vi "DisplayZstack 4 Vicki.vi"(0 "Path":path, 2 "Zplanes":dbl[](array[numeric]), 3 "DAQGain":u16(ring) items=["0.5     +/- 10 V", "1        +/- 5 V", "2.5     +/- 2 V", "5        +/- 1 V", "10      +/- 500 mV", "25      +/- 200 mV", "50      +/- 100 mV"], 5 "Z factor":dbl=161.64 format="%#.2g", 7 "Controls Cluster":T8={"Pockels Control"=0.0, "PMT1"=0, "PMT2"=0, "No of Averages"=0, "Pockels"=0.4817984955602135, "Back Aperture"=19.585304697569654} {"Back Aperture" format="%_2f"; "Pockels" format="%_3g"; "No of Averages" min=0 max=2 step=1 scale=0.0..64.0; "PMT2" min=0 max=1000 step=1 scale=0.0..1000.0; "PMT1" min=0 max=1000 step=1 scale=0.0..1000.0; "Pockels Control" min=0.0 max=2.0 step=0.01 scale=0.0..2.0 scale format="%#4_4f"}, 9 "AOD Parameters":T5={"Nvox"=200, "Zoom"=1, "Xc"=0.0, "Yc"=0.0, "Acceptance Angle"=4.349999904632568, "AOD Central Frequency"=34, "movex"=1.0, "movey"=1.0, "astig"=1.0, "p"=1.0, "Dwell Time"=1.0, "Z Position"=0.0, "xoma"=1.0, "xoda"=1.0, "yoma"=1.0, "yoda"=1.0, "Nx"=0.0, "msReduce"=1.0} {"yoda" min=0.5 max=1.5 step=0.01; "yoma" min=0.5 max=1.5 step=0.01; "xoda" min=0.5 max=1.5 step=0.0005; "xoma" min=0.5 max=1.5 step=0.01; "Z Position" min=-1 max=1 step=0.05 scale=-0.8..0.8 scale format="%#_2g"; "Dwell Time" min=1.0 max=400.0 step=1.0 scale=1.0..400.0; "Nvox" min=10 step=1 scale=10.0..1024.0; "Zoom" min=1 max=10 step=1 scale=1.0..10.0}, 11 "ScanMode":bool, 12 "Pockels Array":dbl[](array[numeric]), 13 "Objective":u16(ring)=1 items=["25X", "40X"], 14 "Field of View":u16(ring) items=["130", "175", "260"]) -> (1 "PMC_Pockels":dbl[](array[numeric]), 4 "output cluster":T4, 6 "TrigDelay(sec) 2":sgl min=0 max=6 step=0.5)   [LabVIEW 2017]
uses:
  <vilib>/vision/Image Controls.llb/IMAQ Image.ctl
  <userlib>/My Palettes.lib/Files & paths/Spreadsheet/Read From Spreadsheet File (string)-Mod.vi
  <userlib>/My Palettes.lib/Files & paths/Spreadsheet/Read From Spreadsheet File (DBL)-Mod.vi
  <vilib>/vision/NI_Vision_Development_Module.lvlib
  <userlib>/My Palettes.lib/Files & paths/Spreadsheet/Write To Spreadsheet File (DBL)-Mod.vi
panel:
  out "Lines":T1(array[cluster]) {"End Point"."Y" format="%.2f"; "End Point"."X" format="%.2f"; "Start Point"."Y" format="%.2f"; "Start Point"."X" format="%.2f"}
  out "most horizontal":T2
  out "most Verital":T2
  out "height":dbl
  out "width":dbl
  out "Number of Files":i32
  out "upper":u16
  out "lower":u16
  out "temp copy":T3
  in  "FilePattern 2":string="Red*"
  in  "FilePattern":string="Green*"
  in  "TrigDelay(sec)":sgl min=0 max=6 step=0.5
  in  "LoadedPOISelect Array":cluster{"System Array":dbl[], "Boolean":bool}[](array[cluster])
  in  "Yoffset":dbl
  in  "Xoffset":dbl
  in  "Z-Offset":dbl
  in  "SaveNotes":bool
  in  "POISelect Array":cluster{"System Array":dbl[], "Boolean":bool}[](array[cluster])
  in  "InvertSelection":bool
  in  "SelectAll":bool
  in  "MaxZproj":bool
  in  "Channel":u16(ring) items=["Red Channel", "Green Channel"]
  in  "TrialDelay":u32=5000 min=3000 max=15000 step=500
  in  "No.ofTrials":dbl=1.0
  out "DwelTime2":i32=4
  in  "DwelTime":u32=1
  in  "Length(msec)":dbl=2000.0
  out "No. of cycles":i32=1
  in  "Nvox":i32=200
  in  "GridNumberZ":i8=1 min=1 step=2
  in  "GridNumberXY":i8=1 min=1 step=2
  in  "LoadPoints":bool
  in  "ClearLast":bool
  in  "ClearAll":bool
  in  "Palette":u16(ring) items=["Gray", "Binary", "Gradient", "Rainbow", "Temperature"]
  in  "stop":bool
  out "RedMaxZ":T3
  in  "LUT1":cluster{u16, u16}(slide)={0, 4095} caption="Slide" scale=0.0..4095.0
  out "Z index 2":dbl
  out "Z Plane":dbl
  in  "Z index":i32(c297)
  out "Image":T3(plugin-control)
  out "DAQRange":dbl
  out "Number of Matches Returned":i32
  in  "Find Lines":bool
  in  "Show Dendrties":bool
  out "Ref Bottom":u16
  out "Ref Right":u16
  out "RefTop":u16
  out "Ref Left":u16
  in  "Boundary":u16
  out "Coordinates":i32[](array[numeric])
  out "Reference Rectangles":dbl[][](array[numeric]) format="%.2f"
  out "Left":dbl
  out "Top":dbl
  out "Right":dbl
  out "Bottom":dbl
  out "Number \nof Particles":i32
  out "Mean Value":sgl format="%.2f"
  out "Histogram Graph":T6 {"Incremental Value" format="%.2f"; "Starting Value" format="%.2f"}
  in  "Show Binary":bool
  out "Reference Screen":T3(plugin-control)
  out "got copy":bool=TRUE
  out "All Files in Dir":path[](array[path])
  out "Global Report":T7 {"Mean Value" format="%.2f"; "%" format="%.2f"; "Area (calibrated)" format="%.2f"; "Maximal Value" format="%.2f"; "Minimal Value" format="%.2f"; "Standard Variation" format="%.2f"}
  in  "Notes":string
  out "NormalizedXYZ":dbl[][](array[numeric])
  in  "Count":i32
  out "POI array":dbl[][](array[numeric])
  out "GreenMaxZ":T3
  out "GreenImageArray":T3[](array[typedef])
  out "RedImageArray":T3[](array[typedef])
  # "POI #"
  # "X"
  # "Y"
  # "Z"
  # "Dwell Time"
  # "msec"
  # "mW"
  # "mW"
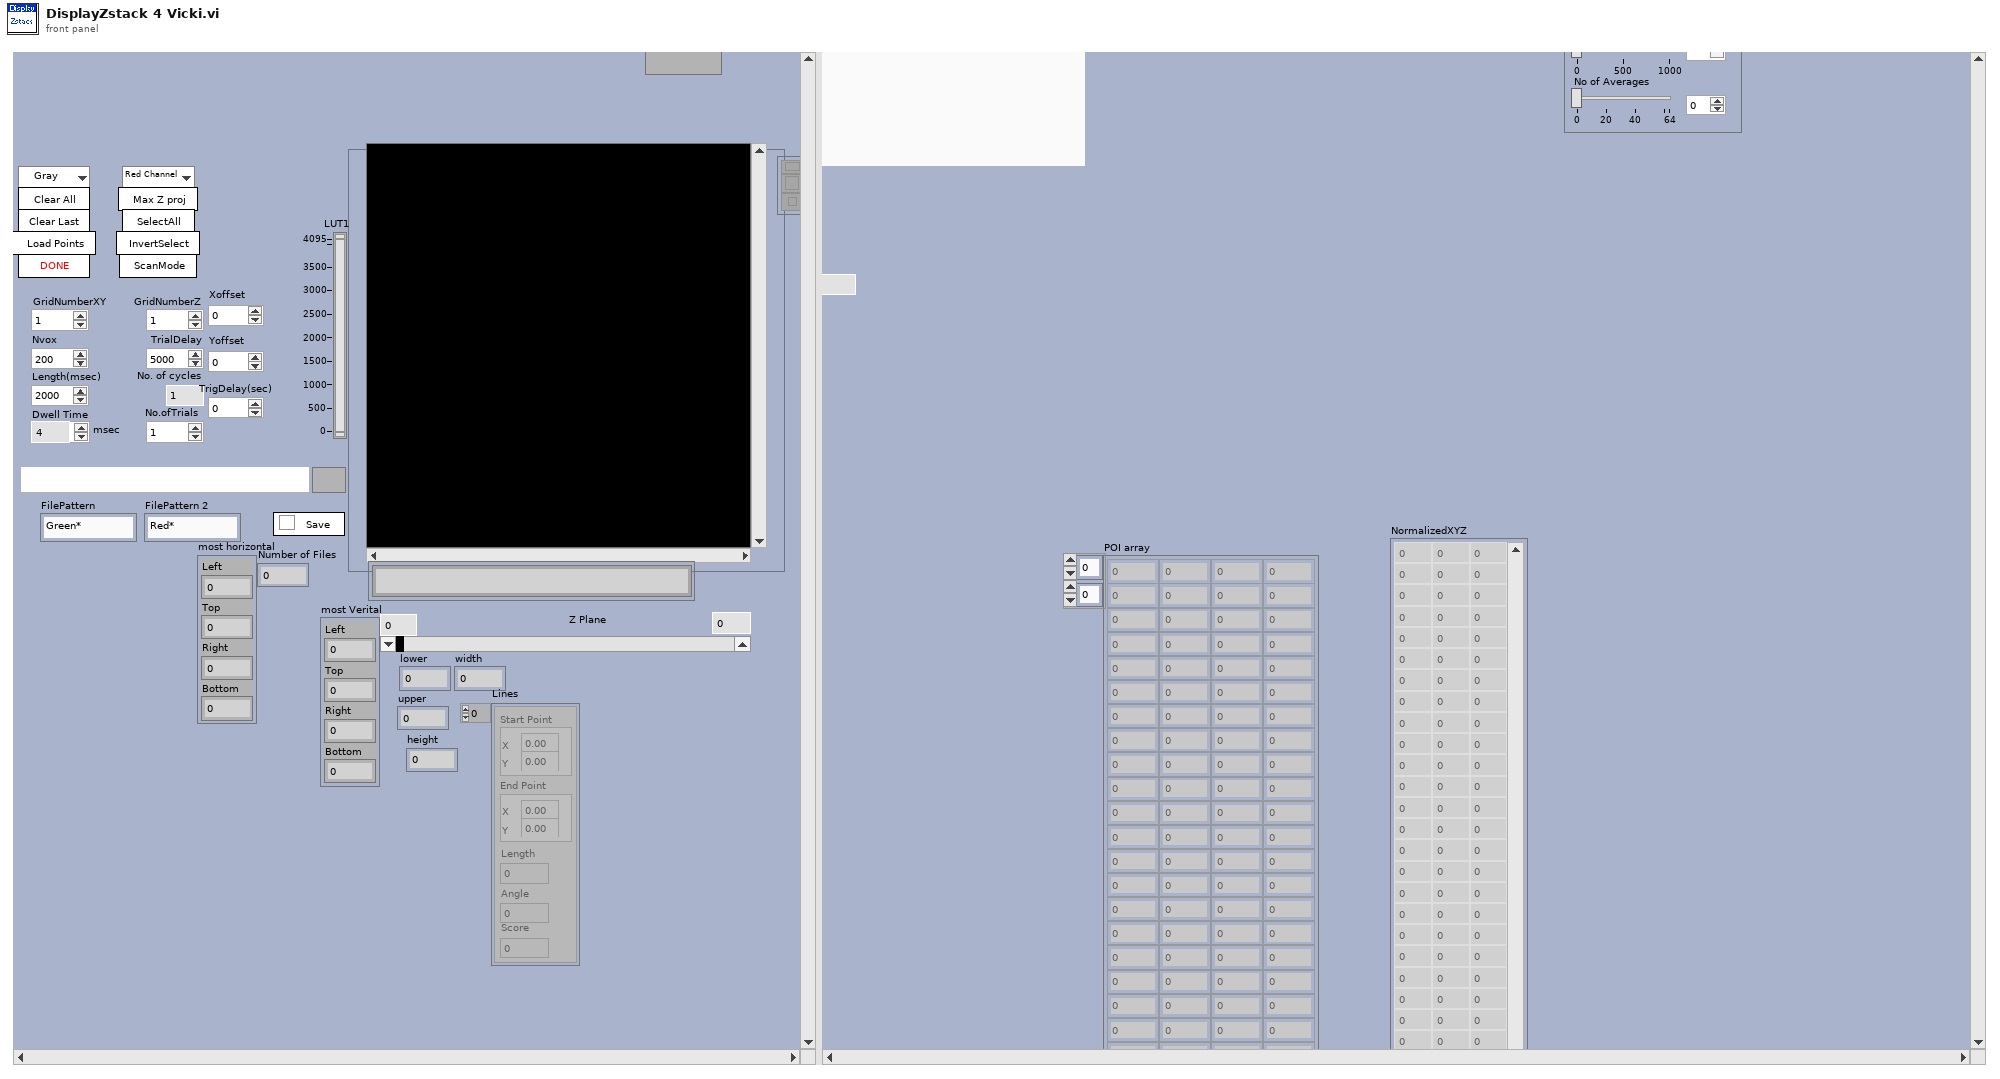
[diagram p1: front panel]
types:
  T1 = cluster{"Start Point":cluster{"X":sgl, "Y":sgl}, "End Point":cluster{"X":sgl, "Y":sgl}, "Length":dbl, "Angle":dbl, "Score":dbl}[]
  T2 = cluster{"Left":i32, "Top":i32, "Right":i32, "Bottom":i32}
  T3 = typedef "IMAQ Image.ctl" = refnum<image>
  T4 = cluster{"xyz coordinates":dbl[][], "Mx offset":dbl, "My offset":dbl, "gridnumberXYout":i8, "gridnumberZout":i8, "NvoxOut":i32, "number of cycles out":i32, "AODfill":dbl, "No. of Trials":dbl, "Dwell Time":i32, "Trial Delay":u32}
  T5 = cluster{"Nvox":i16, "Zoom":i8, "Xc":dbl, "Yc":dbl, "Acceptance Angle":dbl, "AOD Central Frequency":i32, "movex":dbl, "movey":dbl, "astig":dbl, "p":dbl, "Dwell Time":dbl, "Z Position":sgl, "xoma":sgl, "xoda":sgl, "yoma":sgl, "yoda":sgl, "Nx":dbl, "msReduce":dbl}
  T6 = cluster{"Starting Value":sgl, "Incremental Value":sgl, "Histogram":u32[]}
  T7 = cluster{"Mean Value":sgl, "Standard Variation":sgl, "Minimal Value":sgl, "Maximal Value":sgl, "Area (calibrated)":sgl, "Area (pixels)":i32, "%":sgl}
  T8 = cluster{"Pockels Control":dbl, "PMT1":i32, "PMT2":i32, "No of Averages":i32, "Pockels":dbl, "Back Aperture":dbl}
  T9 = enum8{"Enabled", "Disabled", "Disabled and Grayed Out"}
  T10 = typedef "Image Type" = u32
  T11 = enum32{"Average", "Min", "Max", "Clear  if < ", "Clear  if < or =", "Clear  if =", "Clear  if > or =", "Clear  if >"}
  T12 = cluster{"Conversion Method":u32, "Minimum Value":i32, "Maximum Value":i32, "Number Of Shifts":i32}
  T13 = enum16{"open", "replace", "create", "open or create", "replace or create", "replace or create with confirmation"}
  T14 = enum32{"AutoM", "Close", "Dilate", "Erode", "Gradient", "Gradient out", "Gradient in", "Hit miss", "Open", "PClose", "POpen", "Thick", "Thin"}
  T15 = typedef "Particle Parameters" = i32
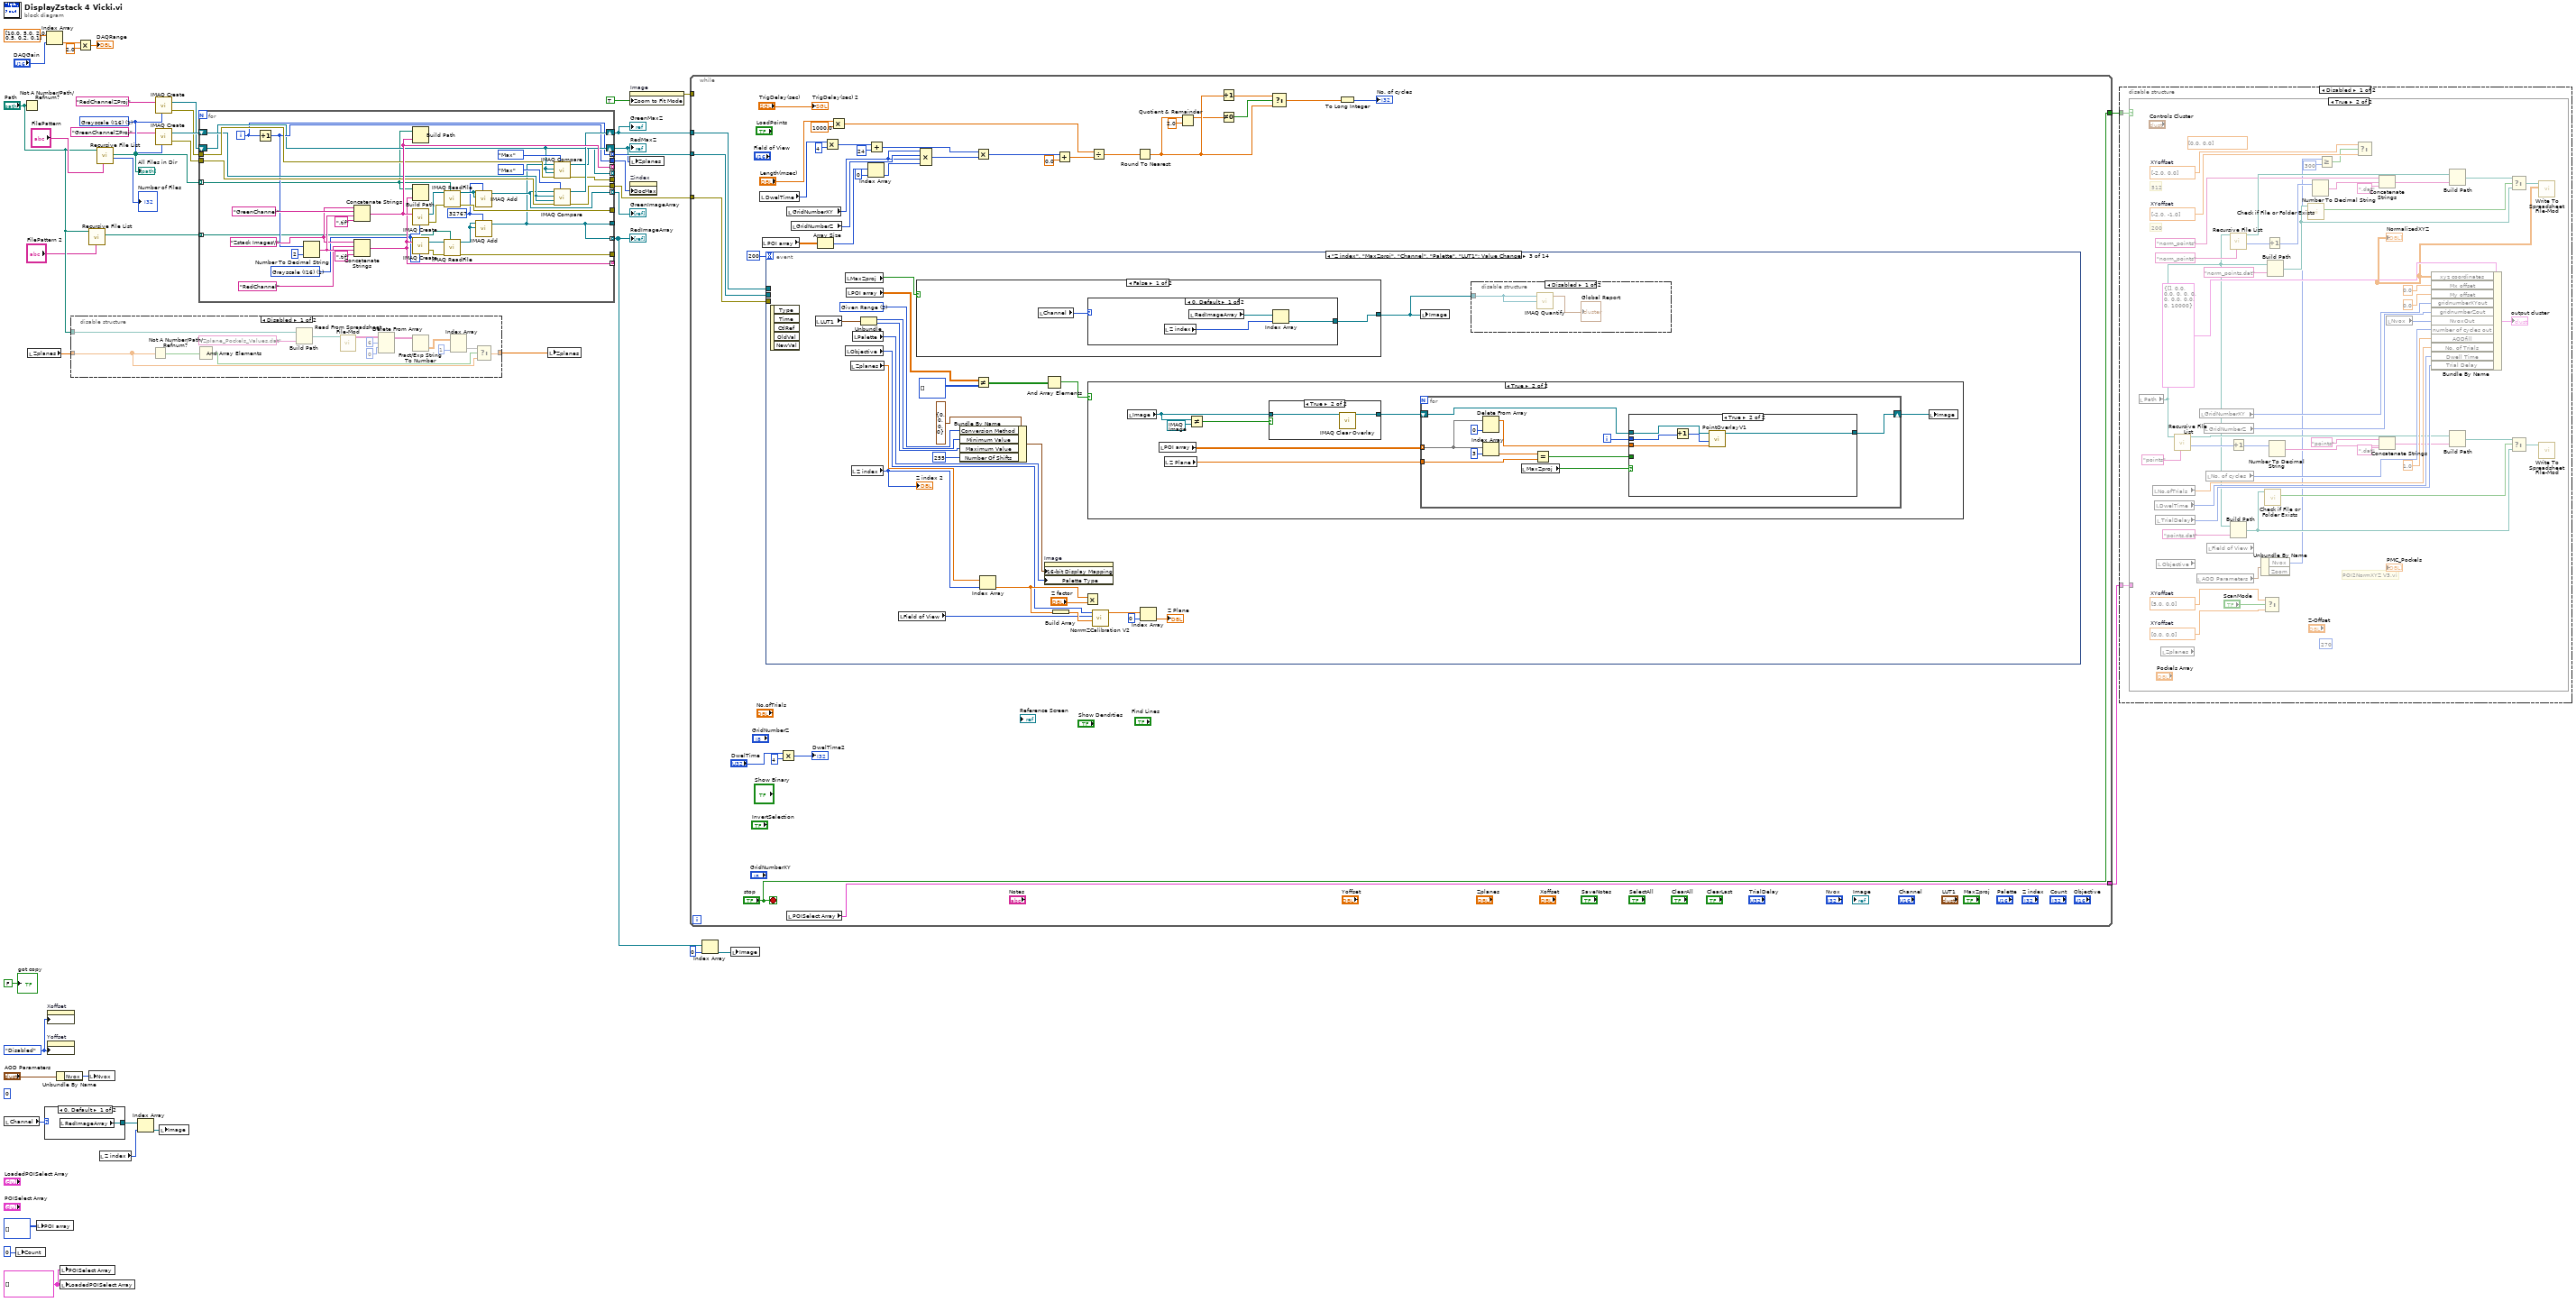
[diagram p0: block diagram]
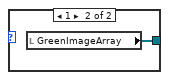
[diagram p5: hidden frame]
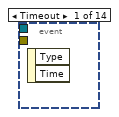
[diagram p6: hidden frame]
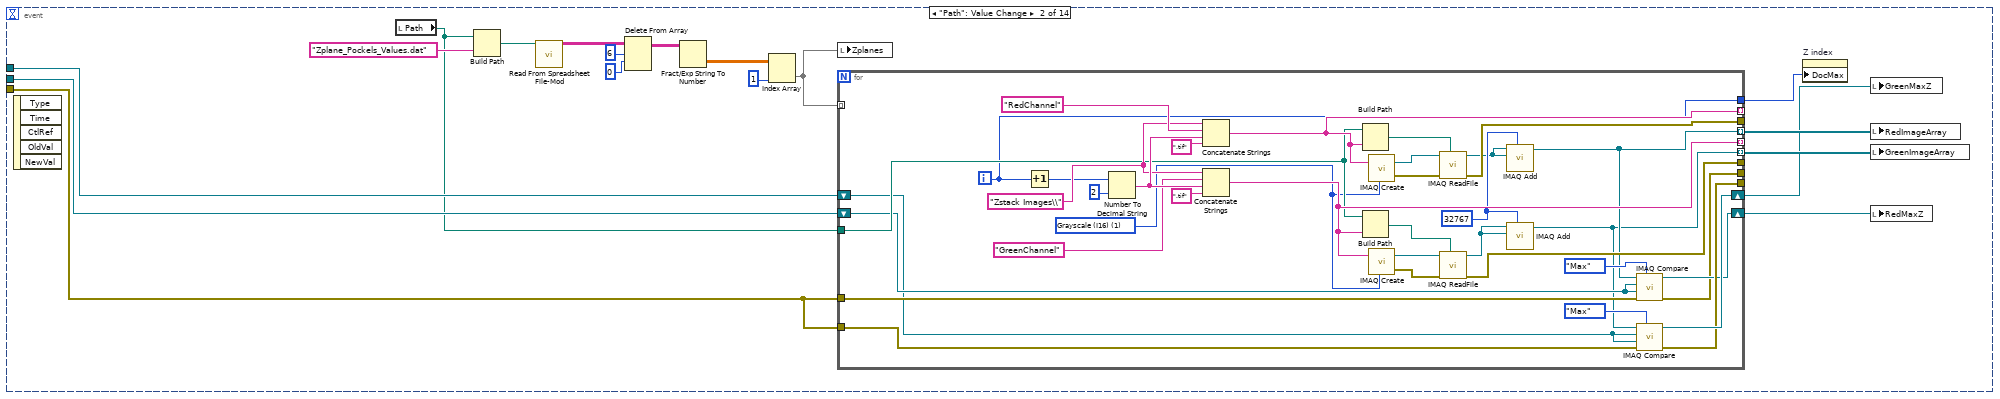
[diagram p7: hidden frame]
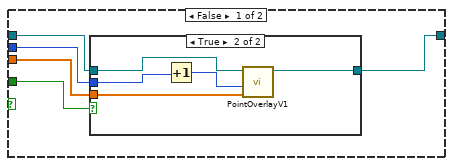
[diagram p11: hidden frame]
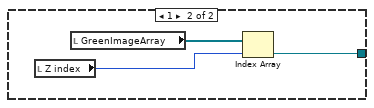
[diagram p13: hidden frame]
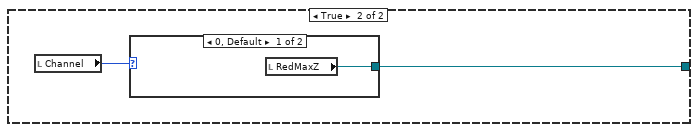
[diagram p14: hidden frame]
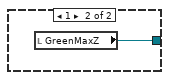
[diagram p15: hidden frame]
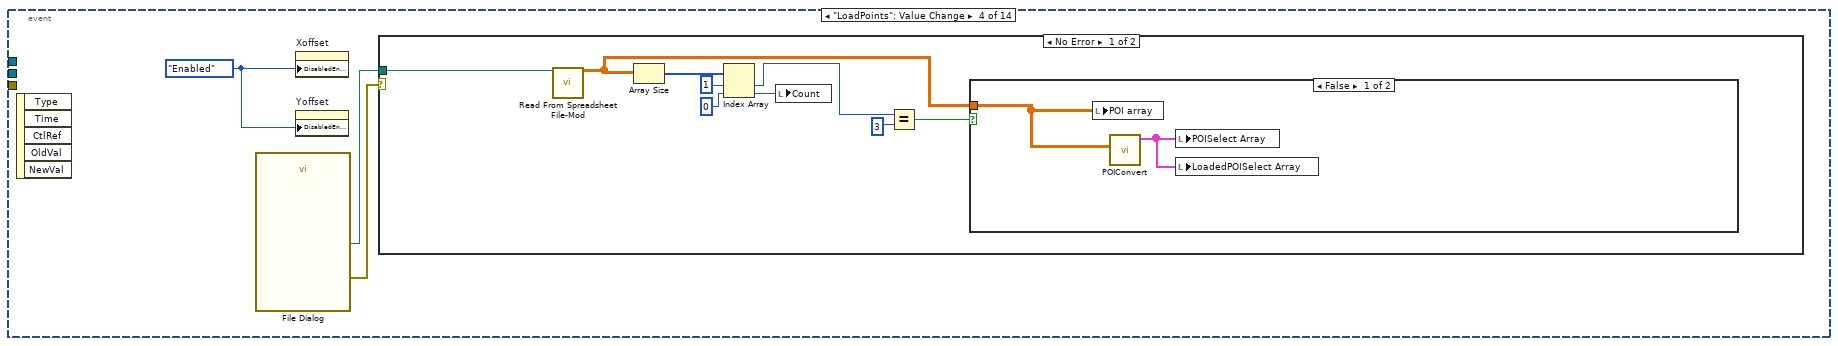
[diagram p16: hidden frame]
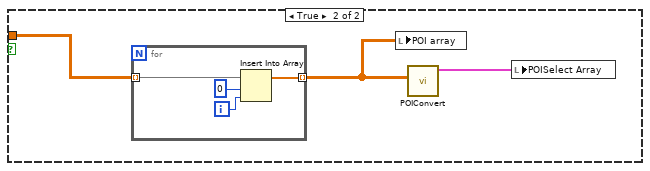
[diagram p17: hidden frame]
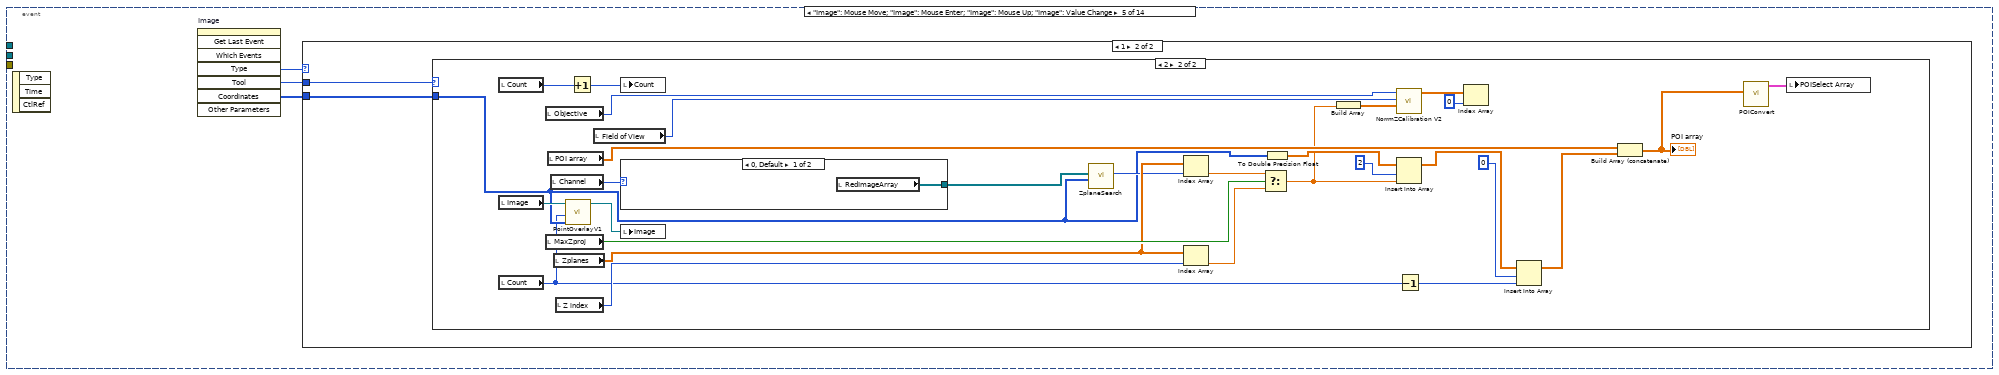
[diagram p19: hidden frame]
diagram:
  w10 = T9."Disabled" ("Disabled")
  (unwired) 0
  w11 = cluster{"System Array":dbl[], "Boolean":bool}[] [] ("POISelect Array")
  w44 = T10 1 items=["Grayscale (U8)", "Grayscale (I16)", "Grayscale (SGL)", "Complex (CSG)", "RGB (U32)", "HSL (U32)", "RGB (U64)"] ("Image Type")
  n1 = local read "Channel"() -> (w32:u16)
  n2 = local write "Count"(0 ("Count")) -> ()
  n3 = Not A Number/Path/Refnum?(number/path/refnum="Path") -> ()  [unwired: 1 out]
  n4 = local read "Zplanes"() -> (w2:dbl[])
  n5 = local write "POI array"(i32[][] [] ("POI array")) -> ()
  n6 = case shown="0, Default" w32 {
    tunnel: [w45 w46] -> w31
    frame 0, Default {
      n7 = local read "RedImageArray"() -> (w45:T3[])
    }
    frame 1 {
      n8 = local read "GreenImageArray"() -> (w46:T3[])
    }
  }
  n9 = Index Array(array=dbl[] [10.0, 5.0, 2.0, 1.0, 0.5, 0.2, 0.1] ("Array"), index="DAQGain") -> (element=w26:dbl)
  n10 = property on="Xoffset" class="DigNum (strict)"("DisabledEnum"=w10) -> ()  [unwired: 2 in, 2 out]
  n11 = property on="Yoffset" class="DigNum (strict)"("DisabledEnum"=w10) -> ()  [unwired: 2 in, 2 out]
  n12 = Unbundle By Name("AOD Parameters") -> ("Nvox"=w16:i16)
  n13 = local write "POISelect Array"(w11) -> ()
  n14 = local write "LoadedPOISelect Array"(w11) -> ()
  n15 = disable-structure shown="Disabled" {
    disable-tunnel: w2 -> [w50 _]
    disable-tunnel: [w49 _] -> w19
    disable-tunnel: "Path" -> [w48 _]
    frame Disabled {
      n16 = Not A Number/Path/Refnum?(number/path/refnum=w50) -> (NaN/Path/Refnum?=w59:bool[])
      n17 = And Array Elements(Boolean array=w59) -> (logical AND=w58:bool)
      n18 = Build Path(base path=w48, name or relative path="Zplane_Pockels_Values.dat") -> (appended path=w51:path)
      n19 = call-poly <userlib>:"Read From Spreadsheet File-Mod.vi"("file path (dialog if empty)"=w51) -> ("all rows"=w47:string[][])  [unwired: 9 in, 5 out]
      n20 = Delete From Array(array=w47, length=6, index (row)=0) -> (array with subset deleted=w55:string[][])  [unwired: 1 in, 1 out]
      n21 = Fract/Exp String To Number(string=w55) -> (number=w54:dbl[][])  [unwired: 3 in, 1 out]
      n22 = Index Array(array=w54, index (col)=1 ("disabled index (col)")) -> (element=w60:dbl[])  [unwired: 1 in]
      n23 = Select(t=w60, s=w58, f=w50) -> (s? t:f=w49:dbl[])
    }
    frame Enabled {
    }
  }
  n24 = Multiply(x=w26, y=2.0) -> (x*y=→"DAQRange":dbl)
  n25 = local write "Nvox"(w16) -> ()
  n26 = call <vilib>:"Recursive File List.vi"("pattern"="FilePattern 2", "Folder Path"="Path") -> ("All Files in Dir"=w4:path[])  [unwired: 5 in, 4 out]
  n27 = call <vilib>:"Recursive File List.vi"("pattern"="FilePattern", "Folder Path"="Path") -> ("Number of Files"=→"Number of Files":i32, "All Files in Dir"=w7:path[])  [unwired: 5 in, 3 out]
  "All Files in Dir" <- w7
  n28 = local read "Z index"() -> (w30:i32)
  n29 = Index Array(array=w31, index=w30) -> (element=w33:T3)
  n30 = call "IMAQ Create"("Image Name"="RedChannelZProj" ("string"), "Image Type"=w44) -> ("New Image"=w39:T3, "error out"=w38:errorcluster)  [unwired: 3 in]
  n31 = call "IMAQ Create"("Image Name"="GreenChannelZProj" ("string"), "Image Type"=w44) -> ("New Image"=w41:T3, "error out"=w40:errorcluster)  [unwired: 3 in]
  n32 = local write "Image"(w33) -> ()
  n33 = for {
    tunnel: [w66] -> w18 mode=indexing
    tunnel: [w67] -> w22 mode=indexing
    tunnel: w7 -> [w62] mode=indexing
    tunnel: [w84] -> _ mode=indexing
    tunnel: [w83] -> _ mode=indexing
    tunnel: [w82] -> _
    tunnel: [w81] -> _
    shift-right: [w80] -> w36
    shift-left: w41 -> [w72]
    tunnel: [w79] -> w37
    tunnel: w40 -> [w78]
    shift-right: [w77] -> w35
    shift-left: w39 -> [w64]
    tunnel: w38 -> [w76]
    tunnel: [w75] -> _
    tunnel: [w65] -> w23
    tunnel: [w66] -> _
    tunnel: [w64] -> _ mode=indexing
    tunnel: w4 -> [w63] mode=indexing
    tunnel: [w61] -> w3 mode=indexing
    i -> [w61]
    w68 = i16 32767 ("Constant")
    w85 = "Zstack Images\\" ("string")
    w71 = T10 1 items=["Grayscale (U8)", "Grayscale (I16)", "Grayscale (SGL)", "Complex (CSG)", "RGB (U32)", "HSL (U32)", "RGB (U64)"] ("Image Type")
    n34 = Increment(x=w61) -> (x+1=w65:i32)
    n35 = Number To Decimal String(number=w65, width (-)=i16 2) -> (decimal integer string=w90:string)
    n36 = Concatenate Strings(w85, "GreenChannel" ("string"), w90, ".tif" ("string")) -> (w84:string)
    n37 = Concatenate Strings(w85, "RedChannel" ("string"), w90, ".tif" ("string")) -> (w83:string)
    n38 = Build Path(base path=w62, name or relative path=w84) -> ()  [unwired: 1 out]
    n39 = Build Path(base path=w62, name or relative path=w83) -> ()  [unwired: 1 out]
    n40 = call "IMAQ Create"("Image Name"=w84, "Image Type"=w71) -> ("New Image"=w93:T3, "error out"=w92:errorcluster)  [unwired: 3 in]
    n41 = call "IMAQ Create"("Image Name"=w83, "Image Type"=w71) -> ("New Image"=w94:T3, "error out"=w95:errorcluster)  [unwired: 3 in]
    n42 = call "IMAQ ReadFile"("File Path"=w62, "error in (no error)"=w92, "Image"=w93) -> ("error out"=w81:errorcluster, "Image Out"=w70:T3)  [unwired: 4 in, 3 out]
    n43 = call "IMAQ ReadFile"("File Path"=w63, "error in (no error)"=w95, "Image"=w94) -> ("error out"=w82:errorcluster, "Image Out"=w69:T3)  [unwired: 4 in, 3 out]
    n44 = call "IMAQ Add"("Image Src A"=w70, "Constant"=w68, "Image Dst"=w70) -> ("Image Dst Out"=w67:T3)  [unwired: 4 in, 1 out]
    n45 = call "IMAQ Add"("Image Src A"=w69, "Constant"=w68, "Image Dst"=w69) -> ("Image Dst Out"=w66:T3)  [unwired: 4 in, 1 out]
    n46 = call "IMAQ Compare"("Operator"=T11."Max", "error in (no error)"=w76, "Image Src B"=w64, "Image Dst"=w64, "Image Src A"=w66) -> ("error out"=w75:errorcluster, "Image Dst Out"=w77:T3)  [unwired: 5 in]
    n47 = call "IMAQ Compare"("Operator"=T11."Max", "error in (no error)"=w78, "Image Src B"=w72, "Image Dst"=w72, "Image Src A"=w67) -> ("error out"=w79:errorcluster, "Image Dst Out"=w80:T3)  [unwired: 5 in]
  }
  "RedImageArray" <- w18
  "GreenImageArray" <- w22
  "RedMaxZ" <- w35
  "GreenMaxZ" <- w36
  n48 = local write "Zplanes"(w19) -> ()
  n49 = property on="Image" class="ImageControl"("Zoom to Fit Mode"=TRUE) -> (error out=w14:errorcluster)  [unwired: 2 in, 1 out]
  n50 = local write "Zplanes"(w3) -> ()
  n51 = property on="Zindex" class="Scroll (strict)"("DocMax"=w23) -> ()  [unwired: 2 in, 2 out]
  n52 = while {
    tunnel: w37 -> [w131]
    tunnel: w35 -> [w130]
    tunnel: w36 -> [w129]
    tunnel: [w124] -> w21
    tunnel: ["stop"] -> w20
    tunnel: w14 -> [_]
    stop <- "stop" stop-if-true
    n53 = local read "DwelTime"() -> (w108:u32)
    n54 = local read "POI array"() -> (w97:dbl[][])
    n55 = event shown="[2] \"Z index\", \"MaxZproj\", \"Channel\", \"Palette\", \"LUT1\": Value Change" {
      selector: _ -> [_ _ _ _ _ _ _ _ _ _ _ _ _ _]
      dyn-events: _ -> [_ _ _ _ _ _ _ _ _ _ _ _ _ _]
      timeout: 200 -> [_ _ _ _ _ _ _ _ _ _ _ _ _ _]
      tunnel: w131 -> [_ w149 _ _ _ _ _ _ _ _ _ _ _ _]
      tunnel: w130 -> [_ w148 _ _ _ _ _ _ _ _ _ _ _ _]
      tunnel: w129 -> [_ w147 _ _ _ _ _ _ _ _ _ _ _ _]
      event Timeout {
        n56 = event-data() -> ()  [unwired: 1 in, 2 out]
      }
      event "Path": Value Change {
        n57 = event-data() -> ()  [unwired: 1 in, 5 out]
        n58 = local read "Path"() -> (w139:path)
        n59 = Build Path(base path=w139, name or relative path="Zplane_Pockels_Values.dat") -> (appended path=w146:path)
        n60 = call-poly <userlib>:"Read From Spreadsheet File-Mod.vi"("file path (dialog if empty)"=w146) -> ("all rows"=w132:string[][])  [unwired: 9 in, 5 out]
        n61 = Delete From Array(array=w132, length=6, index (row)=0) -> (array with subset deleted=w142:string[][])  [unwired: 1 in, 1 out]
        n62 = Fract/Exp String To Number(string=w142) -> (number=w143:dbl[][])  [unwired: 3 in, 1 out]
        n63 = Index Array(array=w143, index (col)=1 ("disabled index (col)")) -> (element=w138:dbl[])  [unwired: 1 in]
        n64 = local write "Zplanes"(w138) -> ()
        n65 = for {
          tunnel: [w153] -> w135 mode=indexing
          tunnel: [w152] -> w136 mode=indexing
          tunnel: w139 -> [w170]
          tunnel: [w172] -> _ mode=indexing
          tunnel: [w171] -> _ mode=indexing
          tunnel: [w169] -> _
          tunnel: [w168] -> _
          shift-right: [w165] -> w134
          shift-left: w147 -> [w156]
          tunnel: [w164] -> _
          tunnel: w149 -> [w163]
          shift-right: [w162] -> w133
          shift-left: w148 -> [w157]
          tunnel: w149 -> [w161]
          tunnel: [w160] -> _
          tunnel: w138 -> [_] mode=indexing
          tunnel: [w150] -> w137
          i -> [w150]
          w167 = i16 32767 ("Constant")
          w173 = "Zstack Images\\" ("string")
          w151 = T10 1 items=["Grayscale (U8)", "Grayscale (I16)", "Grayscale (SGL)", "Complex (CSG)", "RGB (U32)", "HSL (U32)", "RGB (U64)"] ("Image Type")
          n66 = Increment(x=w150) -> (x+1=w166:i32)
          n67 = Number To Decimal String(number=w166, width (-)=i16 2) -> (decimal integer string=w178:string)
          n68 = Concatenate Strings(w173, "RedChannel" ("string"), w178, ".tif" ("string")) -> (w171:string)
          n69 = Concatenate Strings(w173, "GreenChannel" ("string"), w178, ".tif" ("string")) -> (w172:string)
          n70 = Build Path(base path=w170, name or relative path=w171) -> (appended path=w181:path)
          n71 = Build Path(base path=w170, name or relative path=w172) -> (appended path=w180:path)
          n72 = call "IMAQ Create"("Image Name"=w171, "Image Type"=w151) -> ("New Image"=w184:T3, "error out"=w185:errorcluster)  [unwired: 3 in]
          n73 = call "IMAQ Create"("Image Name"=w172, "Image Type"=w151) -> ("New Image"=w183:T3, "error out"=w182:errorcluster)  [unwired: 3 in]
          n74 = call "IMAQ ReadFile"("File Path"=w181, "error in (no error)"=w185, "Image"=w184) -> ("error out"=w169:errorcluster, "Image Out"=w155:T3)  [unwired: 4 in, 3 out]
          n75 = call "IMAQ ReadFile"("File Path"=w180, "error in (no error)"=w182, "Image"=w183) -> ("error out"=w168:errorcluster, "Image Out"=w154:T3)  [unwired: 4 in, 3 out]
          n76 = call "IMAQ Add"("Image Src A"=w155, "Constant"=w167, "Image Dst"=w155) -> ("Image Dst Out"=w153:T3)  [unwired: 4 in, 1 out]
          n77 = call "IMAQ Add"("Image Src A"=w154, "Constant"=w167, "Image Dst"=w154) -> ("Image Dst Out"=w152:T3)  [unwired: 4 in, 1 out]
          n78 = call "IMAQ Compare"("Operator"=T11."Max", "error in (no error)"=w161, "Image Src B"=w157, "Image Dst"=w157, "Image Src A"=w153) -> ("error out"=w160:errorcluster, "Image Dst Out"=w162:T3)  [unwired: 5 in]
          n79 = call "IMAQ Compare"("Operator"=T11."Max", "error in (no error)"=w163, "Image Src B"=w156, "Image Dst"=w156, "Image Src A"=w152) -> ("error out"=w164:errorcluster, "Image Dst Out"=w165:T3)  [unwired: 5 in]
        }
        n80 = property on="Z index" class="Scroll (strict)"("DocMax"=w137) -> ()  [unwired: 2 in, 2 out]
        n81 = local write "GreenMaxZ"(w134) -> ()
        n82 = local write "RedImageArray"(w135) -> ()
        n83 = local write "GreenImageArray"(w136) -> ()
        n84 = local write "RedMaxZ"(w133) -> ()
      }
      event "Z index", "MaxZproj", "Channel", "Palette", "LUT1": Value Change {
        w202 = u32 2 items=["Full Dynamic", "Downshift", "Given Range", "90 % Dynamic", "Given Percent Range"] ("Conversion Method")
        n85 = event-data() -> ()  [unwired: 1 in, 5 out]
        n86 = local read "LUT1"() -> (w205:cluster{u16, u16})
        n87 = local read "MaxZproj"() -> (w207:bool)
        n88 = local read "Objective"() -> (w187:u16)
        n89 = local read "POI array"() -> (w197:dbl[][])
        n90 = local read "Zplanes"() -> (w209:dbl[])
        n91 = local read "Z index"() -> (w206:i32)
        "Z index 2" <- w206
        n92 = local read "Palette"() -> (w198:u16)
        n93 = Unbundle(w205) -> (w204:u16, w203:u16)
        n94 = local read "Field of View"() -> (w186:u16)
        n95 = case shown="False" w207 {
          tunnel: [w249 w257] -> w193
          frame False {
            n96 = local read "Channel"() -> (w250:u16)
            n97 = case shown="0, Default" w250 {
              tunnel: [w251 w254] -> w249
              frame 0, Default {
                n98 = local read "Z index"() -> (w252:i32)
                n99 = local read "RedImageArray"() -> (w253:T3[])
                n100 = Index Array(array=w253, index=w252) -> (element=w251:T3)
              }
              frame 1 {
                n101 = local read "Z index"() -> (w256:i32)
                n102 = local read "GreenImageArray"() -> (w255:T3[])
                n103 = Index Array(array=w255, index=w256) -> (element=w254:T3)
              }
            }
          }
          frame True {
            n104 = local read "Channel"() -> (w258:u16)
            n105 = case shown="0, Default" w258 {
              tunnel: [w259 w260] -> w257
              frame 0, Default {
                n106 = local read "RedMaxZ"() -> (w259:T3)
              }
              frame 1 {
                n107 = local read "GreenMaxZ"() -> (w260:T3)
              }
            }
          }
        }
        n108 = Bundle By Name(cluster=T12 {"Conversion Method"=0, "Minimum Value"=0, "Maximum Value"=0, "Number Of Shifts"=0} ("16-bit Display Mapping:All Elements"), "Conversion Method"=w202, "Minimum Value"=w204, "Maximum Value"=w203, "Number Of Shifts"=255 ("# Shifts")) -> (w199:T12)
        n109 = Not Equal?(x=w197, y=i32[][] []) -> (x != y?=w195:bool[][])
        n110 = Index Array(array=w209, index=w206) -> (element=w188:dbl)
        n111 = property on="Image" class="ImageControl"("16-bit Display Mapping"=w199, "Palette Type"=w198) -> ()  [unwired: 2 in, 2 out]
        n112 = And Array Elements(Boolean array=w195) -> (logical AND=w194:bool)
        n113 = Build Array(w188) -> (w189:dbl[])
        n114 = Multiply(x=w188, y="Z factor") -> ()  [unwired: 1 out]
        n115 = case shown="True" w194 {
          frame False {
          }
          frame True {
            n116 = local read "Image"() -> (w214:T3)
            n117 = local read "POI array"() -> (w216:dbl[][])
            n118 = local read "Z Plane"() -> (w218:dbl)
            n119 = Not Equal?(x=w214, y=T3 refnum) -> (x != y?=w213:bool)
            n120 = case shown="True" w213 {
              tunnel: [w219 w221] -> w212
              tunnel: w214 -> [w219 w220]
              frame False {
              }
              frame True {
                n121 = call "IMAQ Clear Overlay"("Image"=w220) -> ("Image Out"=w221:T3)  [unwired: 9 in, 1 out]
              }
            }
            n122 = for {
              tunnel: w216 -> [w227] mode=indexing
              shift-right: [w231] -> w217
              shift-left: w212 -> [w230]
              tunnel: w218 -> [w223]
              i -> [w229]
              n123 = Delete From Array(array=w227, index=0) -> (array with subset deleted=w228:dbl[])  [unwired: 1 in, 1 out]
              n124 = Index Array(array=w227, index=3) -> (element=w225:dbl)
              n125 = local read "MaxZproj"() -> (w222:bool)
              n126 = Equal?(x=w225, y=w223) -> (x = y?=w224:bool)
              n127 = case shown="True" w222 {
                tunnel: [w237 w247] -> w231
                tunnel: w230 -> [w236 w246]
                tunnel: w229 -> [w235 w245]
                tunnel: w228 -> [w234 w244]
                tunnel: w224 -> [w233 _]
                frame False {
                  n128 = case shown="True" w233 {
                    tunnel: [w238 w243] -> w237
                    tunnel: w236 -> [w238 w242]
                    tunnel: w235 -> [_ w241]
                    tunnel: w234 -> [_ w239]
                    frame False {
                    }
                    frame True {
                      n129 = Increment(x=w241) -> (x+1=w240:i32)
                      n130 = call "PointOverlayV1.vi"("Point"=w239, "Count"=w240, "Image1"=w242) -> ("Image1 Out"=w243:T3)  [unwired: 8 in]
                    }
                  }
                }
                frame True {
                  n131 = Increment(x=w245) -> (x+1=w248:i32)
                  n132 = call "PointOverlayV1.vi"("Point"=w244, "Count"=w248, "Image1"=w246) -> ("Image1 Out"=w247:T3)  [unwired: 8 in]
                }
              }
            }
            n133 = local write "Image"(w217) -> ()
          }
        }
        n134 = call "NorrmZCalibration V2.vi"("xi"=w189, "Field of View"=w186, "Objective"=w187) -> ("yi"=w192:dbl[])  [unwired: 6 in, 2 out]
        n135 = Index Array(array=w192, index=0) -> (element=→"Z Plane":dbl)
        n136 = local write "Image"(w193) -> ()
        n137 = disable-structure shown="Disabled" {
          disable-tunnel: w193 -> [w210 _]
          frame Disabled {
            n138 = call "IMAQ Quantify"("Image Mask"=w210, "Image"=w210) -> ("Global Report"=→"Global Report":T7)  [unwired: 1 in, 2 out]
          }
          frame Enabled {
          }
        }
      }
      event "LoadPoints": Value Change {
        w261 = T9."Enabled" ("Disabled")
        n139 = event-data() -> ()  [unwired: 1 in, 5 out]
        n140 = call "File Dialog"() -> ("selected path"=w263:path, "error out"=w262:errorcluster)  [unwired: 12 in, 2 out]
        n141 = property on="Xoffset" class="DigNum (strict)"("DisabledEnum"=w261) -> ()  [unwired: 2 in, 2 out]
        n142 = property on="Yoffset" class="DigNum (strict)"("DisabledEnum"=w261) -> ()  [unwired: 2 in, 2 out]
        n143 = case shown="No Error" w262 {
          tunnel: w263 -> [w272 _]
          frame No Error {
            n144 = call-poly <userlib>:"Read From Spreadsheet File-Mod.vi"("file path (dialog if empty)"=w272) -> ("all rows"=w266:dbl[][])  [unwired: 9 in, 5 out]
            n145 = Array Size(array=w266) -> (size(s)=w271:i32[])
            n146 = Index Array(array=w271, index #1=1 ("index"), index #2=0 ("index")) -> (element #1=w269:i32, element #2=w264:i32)
            n147 = local write "Count"(w264) -> ()
            n148 = Equal?(x=w269, y=3) -> (x = y?=w267:bool)
            n149 = case shown="False" w267 {
              tunnel: w266 -> [w274 w277]
              frame False {
                n150 = local write "POI array"(w274) -> ()
                n151 = call "POIConvert.vi"("POI array"=w274) -> ("POISelectArrayOut"=w273:cluster{"System Array":dbl[], "Boolean":bool}[])  [unwired: 10 in]
                n152 = local write "POISelect Array"(w273) -> ()
                n153 = local write "LoadedPOISelect Array"(w273) -> ()
              }
              frame True {
                n154 = for {
                  tunnel: w277 -> [w281] mode=indexing
                  tunnel: [w278] -> w275 mode=indexing
                  i -> [w280]
                  n155 = Insert Into Array(array=w281, index=0, new element=w280) -> (w278:dbl[])
                }
                n156 = local write "POI array"(w275) -> ()
                n157 = call "POIConvert.vi"("POI array"=w275) -> ("POISelectArrayOut"=w276:cluster{"System Array":dbl[], "Boolean":bool}[])  [unwired: 10 in]
                n158 = local write "POISelect Array"(w276) -> ()
              }
            }
          }
          frame Error {
          }
        }
      }
      event "Image": Mouse Move; "Image": Mouse Enter; "Image": Mouse Up; "Image": Value Change {
        n159 = event-data() -> ()  [unwired: 1 in, 3 out]
        n160 = invoke on="Image" class="ImageControl" method="Get Last Event"() -> ("Type"=w284:i32, "Tool"=w283:i32, "Coordinates"=w282:i32[])  [unwired: 8 in, 5 out]
        n161 = case shown="1" w284 {
          tunnel: w283 -> [_ w286]
          tunnel: w282 -> [_ w285]
          frame 0, Default {
          }
          frame 1 {
            n162 = case shown="2" w286 {
              tunnel: w285 -> [_ w297]
              frame 0, Default {
              }
              frame 2 {
                n163 = local read "Count"() -> (w302:i32)
                n164 = local read "Image"() -> (w300:T3)
                n165 = local read "Count"() -> (w296:i32)
                n166 = local read "Objective"() -> (w292:u16)
                n167 = local read "MaxZproj"() -> (w312:bool)
                n168 = local read "POI array"() -> (w315:dbl[][])
                n169 = local read "Channel"() -> (w307:u16)
                n170 = local read "Zplanes"() -> (w311:dbl[])
                n171 = local read "Z index"() -> (w313:i32)
                n172 = call "PointOverlayV1.vi"("Point"=w297, "Count"=w296, "Image1"=w300) -> ("Image1 Out"=w299:T3)  [unwired: 8 in]
                n173 = Increment(x=w302) -> (x+1=w301:i32)
                n174 = local read "Field of View"() -> (w293:u16)
                n175 = local write "Count"(w301) -> ()
                n176 = case shown="0, Default" w307 {
                  tunnel: [w316 w317] -> w306
                  frame 0, Default {
                    n177 = local read "RedImageArray"() -> (w316:T3[])
                  }
                  frame 1 {
                    n178 = local read "GreenImageArray"() -> (w317:T3[])
                  }
                }
                n179 = local write "Image"(w299) -> ()
                n180 = call "ZplaneSearch.vi"("POI"=w297, "ImageArray"=w306) -> ("ZplaneIndex"=w310:i32)  [unwired: 8 in, 1 out]
                n181 = Index Array(array=w311, index=w310) -> (element=w309:dbl)
                n182 = Index Array(array=w311, index=w313) -> (element=w308:dbl)
                n183 = Select(t=w309, s=w312, f=w308) -> (s? t:f=w287:dbl)
                n184 = To Double Precision Float(number=w297) -> (double precision float=w288:dbl[])
                n185 = Build Array(w287) -> (w291:dbl[])
                n186 = call "NorrmZCalibration V2.vi"("xi"=w291, "Field of View"=w293, "Objective"=w292) -> ("yi"=w289:dbl[])  [unwired: 6 in, 2 out]
                n187 = Insert Into Array(array=w288, index=2, new element=w287) -> (w305:dbl[])
                n188 = Decrement(x=w296) -> (x-1=w298:i32)
                n189 = Index Array(array=w289, index=0) -> ()  [unwired: 1 out]
                n190 = Insert Into Array(array=w305, index=0, new element=w298) -> (w303:dbl[])
                n191 = Build Array (concatenate)(w315, w303) -> (w295:dbl[][])
                "POI array" <- w295
                n192 = call "POIConvert.vi"("POI array"=w295) -> ("POISelectArrayOut"=w294:cluster{"System Array":dbl[], "Boolean":bool}[])  [unwired: 10 in]
                n193 = local write "POISelect Array"(w294) -> ()
              }
            }
          }
        }
      }
      event "ClearAll", "ClearLast": Value Change {
        w318 = T9."Disabled" ("Disabled")
        n194 = event-data() -> ()  [unwired: 1 in, 5 out]
        n195 = local read "ClearLast"() -> (w319:bool)
        n196 = local read "ClearAll"() -> (w320:bool)
        n197 = property on="Xoffset" class="DigNum (strict)"("DisabledEnum"=w318) -> ()  [unwired: 2 in, 2 out]
        n198 = property on="Yoffset" class="DigNum (strict)"("DisabledEnum"=w318) -> ()  [unwired: 2 in, 2 out]
        n199 = case shown="True" w320 {
          frame False {
          }
          frame True {
            w363 = cluster{"System Array":dbl[], "Boolean":bool}[] [] ("POISelect Array")
            n200 = local write "Count"(0 ("Count")) -> ()
            n201 = local read "Image"() -> (w364:T3)
            n202 = local write "POI array"(dbl[][] [] ("POI array")) -> ()
            n203 = call "IMAQ Clear Overlay"("Image"=w364) -> ("Image Out"=w365:T3)  [unwired: 9 in, 1 out]
            n204 = local write "Image"(w365) -> ()
            n205 = local write "POISelect Array"(w363) -> ()
            n206 = local write "LoadedPOISelect Array"(w363) -> ()
          }
        }
        n207 = case shown="True" w319 {
          frame False {
          }
          frame True {
            n208 = local read "Count"() -> (w329:i32)
            n209 = local read "Image"() -> (w327:T3)
            n210 = local read "POI array"() -> (w335:dbl[][])
            n211 = local read "Z Plane"() -> (w323:dbl)
            n212 = Decrement(x=w329) -> (x-1=w328:i32)
            n213 = call "IMAQ Clear Overlay"("Image"=w327) -> ("Image Out"=w326:T3)  [unwired: 9 in, 1 out]
            n214 = local write "Count"(w328) -> ()
            n215 = local write "Image"(w326) -> ()
            n216 = Array Size(array=w335) -> (size(s)=w334:i32[])
            n217 = Index Array(array=w334, index=0) -> (element=w332:i32)
            n218 = Decrement(x=w332) -> (x-1=w330:i32)
            n219 = Delete From Array(array=w335, length=1, index (row)=w330) -> (array with subset deleted=w321:dbl[][])  [unwired: 1 in, 1 out]
            n220 = local write "POI array"(w321) -> ()
            n221 = local read "Image"() -> (w325:T3)
            n222 = call "POIConvert.vi"("POI array"=w321) -> ("POISelectArrayOut"=w322:cluster{"System Array":dbl[], "Boolean":bool}[])  [unwired: 10 in]
            n223 = local write "POISelect Array"(w322) -> ()
            n224 = for {
              tunnel: w321 -> [w341] mode=indexing
              shift-right: [w345] -> w324
              shift-left: w325 -> [w344]
              tunnel: w323 -> [w337]
              i -> [w343]
              n225 = Index Array(array=w341, index=3) -> (element=w339:dbl)
              n226 = Delete From Array(array=w341, index=0) -> (array with subset deleted=w342:dbl[])  [unwired: 1 in, 1 out]
              n227 = local read "MaxZproj"() -> (w336:bool)
              n228 = Equal?(x=w339, y=w337) -> (x = y?=w338:bool)
              n229 = case shown="False" w336 {
                tunnel: [w351 w361] -> w345
                tunnel: w344 -> [w350 w360]
                tunnel: w343 -> [w349 w359]
                tunnel: w342 -> [w348 w358]
                tunnel: w338 -> [w347 _]
                frame False {
                  n230 = case shown="True" w347 {
                    tunnel: [w352 w357] -> w351
                    tunnel: w350 -> [w352 w356]
                    tunnel: w349 -> [_ w355]
                    tunnel: w348 -> [_ w353]
                    frame False {
                    }
                    frame True {
                      n231 = Increment(x=w355) -> (x+1=w354:i32)
                      n232 = call "PointOverlayV1.vi"("Point"=w353, "Count"=w354, "Image1"=w356) -> ("Image1 Out"=w357:T3)  [unwired: 8 in]
                    }
                  }
                }
                frame True {
                  n233 = Increment(x=w359) -> (x+1=w362:i32)
                  n234 = call "PointOverlayV1.vi"("Point"=w358, "Count"=w362, "Image1"=w360) -> ("Image1 Out"=w361:T3)  [unwired: 8 in]
                }
              }
            }
            n235 = local write "Image"(w324) -> ()
          }
        }
      }
      event "SelectAll", "InvertSelection": Value Change {
        n236 = event-data() -> ()  [unwired: 1 in, 5 out]
        n237 = local read "SelectAll"() -> (w368:bool)
        n238 = local read "InvertSelection"() -> (w369:bool)
        n239 = case shown="True" w368 {
          selector: w368 -> [_ w370]
          frame False {
          }
          frame True {
            n240 = local read "Image"() -> (w380:T3)
            n241 = local read "Z Plane"() -> (w376:dbl)
            n242 = call "IMAQ Clear Overlay"("Image"=w380) -> ("error out"=w375:errorcluster, "Image Out"=w379:T3)  [unwired: 9 in]
            n243 = local read "POISelect Array"() -> (w374:cluster{"System Array":dbl[], "Boolean":bool}[])
            n244 = local read "POISelect Array"() -> (w372:cluster{"System Array":dbl[], "Boolean":bool}[])
            n245 = local write "Image"(w379) -> ()
            n246 = call "POISelection.vi"("POISelectArrayIn"=w374) -> ("POI array"=w373:dbl[][])  [unwired: 9 in, 1 out]
            n247 = call "POISelection.vi"("SelectAll"=w370, "POISelectArrayIn"=w372) -> ("POISelectArrayOut"=w371:cluster{"System Array":i32[], "Boolean":bool}[])  [unwired: 8 in, 1 out]
            n248 = local read "Image"() -> (w378:T3)
            n249 = local write "POISelect Array"(w371) -> ()
            n250 = for {
              tunnel: w373 -> [w387] mode=indexing
              shift-right: [w391] -> w377
              shift-left: w378 -> [w390]
              tunnel: w376 -> [w383]
              tunnel: w375 -> [_]
              i -> [w389]
              n251 = Index Array(array=w387, index=3) -> (element=w385:dbl)
              n252 = local read "MaxZproj"() -> (w382:bool)
              n253 = Equal?(x=w385, y=w383) -> (x = y?=w384:bool)
              n254 = Delete From Array(array=w387, index=0) -> (deleted portion=w381:dbl, array with subset deleted=w388:dbl[])  [unwired: 1 in]
              n255 = case shown="True" w382 {
                tunnel: [w397 w408] -> w391
                tunnel: w390 -> [w396 w407]
                tunnel: w389 -> [w395 _]
                tunnel: w388 -> [w394 w406]
                tunnel: w384 -> [w393 _]
                tunnel: w381 -> [_ w405]
                frame False {
                  n256 = case shown="True" w393 {
                    tunnel: [w398 w403] -> w397
                    tunnel: w396 -> [w398 w402]
                    tunnel: w395 -> [_ w401]
                    tunnel: w394 -> [_ w399]
                    frame False {
                    }
                    frame True {
                      n257 = Increment(x=w401) -> (x+1=w400:i32)
                      n258 = call "PointOverlayV1.vi"("Point"=w399, "Count"=w400, "Image1"=w402) -> ("Image1 Out"=w403:T3)  [unwired: 8 in]
                    }
                  }
                }
                frame True {
                  n259 = Increment(x=w405) -> (x+1=w404:dbl)
                  n260 = call "PointOverlayV1.vi"("Point"=w406, "Count"=w404, "Image1"=w407) -> ("Image1 Out"=w408:T3)  [unwired: 8 in]
                }
              }
            }
            n261 = local write "Image"(w377) -> ()
          }
        }
        n262 = case shown="True" w369 {
          selector: w369 -> [_ w409]
          frame False {
          }
          frame True {
            n263 = local read "Image"() -> (w413:T3)
            n264 = call "IMAQ Clear Overlay"("Image"=w413) -> ("Image Out"=w412:T3)  [unwired: 9 in, 1 out]
            n265 = local read "POISelect Array"() -> (w410:cluster{"System Array":dbl[], "Boolean":bool}[])
            n266 = local write "Image"(w412) -> ()
            n267 = call "POISelection.vi"("InvertSelection"=w409, "POISelectArrayIn"=w410) -> ("POISelectArrayOut"=w411:cluster{"System Array":i32[], "Boolean":bool}[])  [unwired: 8 in, 1 out]
            n268 = local write "POISelect Array"(w411) -> ()
          }
        }
      }
      event "POISelect Array": Value Change {
        n269 = event-data() -> ()  [unwired: 1 in, 5 out]
        n270 = local read "Image"() -> (w421:T3)
        n271 = local read "Z Plane"() -> (w417:dbl)
        n272 = call "IMAQ Clear Overlay"("Image"=w421) -> ("error out"=w416:errorcluster, "Image Out"=w420:T3)  [unwired: 9 in]
        n273 = local read "POISelect Array"() -> (w415:cluster{"System Array":dbl[], "Boolean":bool}[])
        n274 = local write "Image"(w420) -> ()
        n275 = call "POISelection.vi"("POISelectArrayIn"=w415) -> ("POI array"=w414:dbl[][])  [unwired: 9 in, 1 out]
        n276 = local read "Image"() -> (w419:T3)
        n277 = for {
          tunnel: w414 -> [w428] mode=indexing
          shift-right: [w431] -> w418
          shift-left: w419 -> [w430]
          tunnel: w417 -> [w424]
          tunnel: w416 -> [_]
          n278 = Index Array(array=w428, index=3) -> (element=w426:dbl)
          n279 = local read "MaxZproj"() -> (w423:bool)
          n280 = Equal?(x=w426, y=w424) -> (x = y?=w425:bool)
          n281 = Delete From Array(array=w428, index=0) -> (deleted portion=w422:dbl, array with subset deleted=w429:dbl[])  [unwired: 1 in]
          n282 = case shown="False" w423 {
            tunnel: [w437 w448] -> w431
            tunnel: w430 -> [w436 w447]
            tunnel: w429 -> [w435 w446]
            tunnel: w425 -> [w434 _]
            tunnel: w422 -> [w433 w445]
            frame False {
              n283 = case shown="True" w434 {
                tunnel: [w438 w443] -> w437
                tunnel: w436 -> [w438 w442]
                tunnel: w433 -> [_ w441]
                tunnel: w435 -> [_ w439]
                frame False {
                }
                frame True {
                  n284 = Increment(x=w441) -> (x+1=w440:dbl)
                  n285 = call "PointOverlayV1.vi"("Point"=w439, "Count"=w440, "Image1"=w442) -> ("Image1 Out"=w443:T3)  [unwired: 8 in]
                }
              }
            }
            frame True {
              n286 = Increment(x=w445) -> (x+1=w444:dbl)
              n287 = call "PointOverlayV1.vi"("Point"=w446, "Count"=w444, "Image1"=w447) -> ("Image1 Out"=w448:T3)  [unwired: 8 in]
            }
          }
        }
        n288 = local write "Image"(w418) -> ()
      }
      event "SaveNotes": Value Change {
        n289 = event-data() -> ()  [unwired: 1 in, 5 out]
        n290 = local read "SaveNotes"() -> (w450:bool)
        n291 = local read "Notes"() -> (w449:string)
        n292 = case shown="True" w450 {
          tunnel: w449 -> [_ w452]
          frame False {
          }
          frame True {
            n293 = Open/Create/Replace File(operation (0:open)=T13."open or create") -> (refnum out=w454:refnum<file>, error out=w453:errorcluster)  [unwired: 5 in, 1 out]
            n294 = Write to Text File(file (use dialog)=w454, text=w452, error in=w453) -> (refnum out=w456:refnum<file>, error out=w455:errorcluster)  [unwired: 1 in, 1 out]
            n295 = Close File(refnum=w456, error in=w455) -> ()  [unwired: 2 out]
          }
        }
      }
      event "Xoffset", "Yoffset": Value Change {
        n296 = event-data() -> ()  [unwired: 1 in, 5 out]
        n297 = local read "POISelect Array"() -> (w459:cluster{"System Array":dbl[], "Boolean":bool}[])
        n298 = local read "LoadedPOISelect Array"() -> (w458:cluster{"System Array":dbl[], "Boolean":bool}[])
        n299 = Empty Array?(array=w458) -> (empty?=w457:bool)
        n300 = case shown="False" w457 {
          selector: w457 -> [_ w510]
          tunnel: w457 -> [w468 _]
          tunnel: w459 -> [w467 _]
          tunnel: w458 -> [w466 _]
          frame False {
            n301 = local read "Image"() -> (w475:T3)
            n302 = Select(t=w467, s=w468, f=w466) -> (s? t:f=w465:cluster{"System Array":dbl[], "Boolean":bool}[])
            n303 = local read "Z Plane"() -> (w471:dbl)
            n304 = local read "Xoffset"() -> (w482:dbl)
            n305 = local read "Yoffset"() -> (w462:dbl)
            n306 = call "POISelection.vi"("POISelectArrayIn"=w465) -> ("POI array"=w480:dbl[][])  [unwired: 9 in, 1 out]
            n307 = call "IMAQ Clear Overlay"("Image"=w475) -> ("error out"=w470:errorcluster, "Image Out"=w474:T3)  [unwired: 9 in]
            n308 = local write "Image"(w474) -> ()
            n309 = Index Array(array=w480, index (col) #1=1 ("index (row)"), index (col) #2=2 ("index (col)")) -> (element #1=w481:dbl[], element #2=w463:dbl[])  [unwired: 2 in]
            n310 = Add(x=w481, y=w482) -> (x+y=w479:dbl[])
            n311 = Add(x=w463, y=w462) -> (x+y=w461:dbl[])
            n312 = Replace Array Subset(array=w480, new element #1=w479, index (col) #1=1 ("disabled index (col)"), new element #2=w461, index (col) #2=2 ("index (col)")) -> (w469:dbl[][])  [unwired: 2 in]
            n313 = local read "Image"() -> (w473:T3)
            n314 = call "POIConvert.vi"("POI array"=w469) -> ("POISelectArrayOut"=w478:cluster{"System Array":dbl[], "Boolean":bool}[])  [unwired: 10 in]
            n315 = local write "POISelect Array"(w478) -> ()
            n316 = for {
              tunnel: w469 -> [w489] mode=indexing
              shift-right: [w492] -> w472
              shift-left: w473 -> [w491]
              tunnel: w471 -> [w485]
              tunnel: w470 -> [_]
              n317 = Index Array(array=w489, index=3) -> (element=w487:dbl)
              n318 = local read "MaxZproj"() -> (w484:bool)
              n319 = Equal?(x=w487, y=w485) -> (x = y?=w486:bool)
              n320 = Delete From Array(array=w489, index=0) -> (deleted portion=w483:dbl, array with subset deleted=w490:dbl[])  [unwired: 1 in]
              n321 = case shown="False" w484 {
                tunnel: [w498 w509] -> w492
                tunnel: w491 -> [w497 w508]
                tunnel: w490 -> [w496 w507]
                tunnel: w486 -> [w495 _]
                tunnel: w483 -> [w494 w506]
                frame False {
                  n322 = case shown="True" w495 {
                    tunnel: [w499 w504] -> w498
                    tunnel: w497 -> [w499 w503]
                    tunnel: w494 -> [_ w502]
                    tunnel: w496 -> [_ w500]
                    frame False {
                    }
                    frame True {
                      n323 = Increment(x=w502) -> (x+1=w501:dbl)
                      n324 = call "PointOverlayV1.vi"("Point"=w500, "Count"=w501, "Image1"=w503) -> ("Image1 Out"=w504:T3)  [unwired: 8 in]
                    }
                  }
                }
                frame True {
                  n325 = Increment(x=w506) -> (x+1=w505:dbl)
                  n326 = call "PointOverlayV1.vi"("Point"=w507, "Count"=w505, "Image1"=w508) -> ("Image1 Out"=w509:T3)  [unwired: 8 in]
                }
              }
            }
            n327 = local write "Image"(w472) -> ()
          }
          frame True {
            w511 = 0.0 ("Yoffset")
            n328 = call "Display Message to User"("Enable"=w510) -> ()  [unwired: 9 in, 2 out]
            n329 = local write "Xoffset"(w511) -> ()
            n330 = local write "Yoffset"(w511) -> ()
          }
        }
      }
      event "Show Binary": Value Change {
        n331 = event-data() -> ()  [unwired: 1 in, 5 out]
        n332 = local read "Show Binary"() -> (w512:bool)
        n333 = case shown="True" w512 {
          frame False {
            n334 = local read "Reference Screen"() -> (w514:T3)
            n335 = call "IMAQ Clear Overlay"("Image"=w514) -> ("error out"=w513:errorcluster)  [unwired: 9 in, 1 out]
            n336 = invoke on="Reference Screen" class="ImageControl" method="Clear ROI"(error in=w513) -> ()  [unwired: 2 in, 3 out]
          }
          frame True {
            w516 = u32 1 items=["Grayscale", "Binary", "Gradient", "Rainbow", "Temperature", "User Defined"] ("Palette:Palette Type")
            w525 = T15[] [4, 5, 6, 7] items=["Center of Mass X", "Center of Mass Y", "First Pixel X", "First Pixel Y", "Bounding Rect Left", "Bounding Rect Top", "Bounding Rect Right", "Bounding Rect Bottom", "Max Feret Diameter Start X", "Max Feret Diameter Start Y", "Max Feret Diameter End X", "Max Feret Diameter End Y", "Max Horiz. Segment Length Left", "Max Horiz. Segment Length Right", "Max Horiz. Segment Length Row", "-", "Bounding Rect Width", "Bounding Rect Height", "Bounding Rect Diagonal", "Perimeter", "Convex Hull Perimeter", "Holes' Perimeter", "Max Feret Diameter", "Equivalent Ellipse Major Axis", "Equivalent Ellipse Minor Axis", "Equivalent Ellipse Minor Axis (Feret)", "Equivalent Rect Long Side", "Equivalent Rect Short Side", "Equivalent Rect Diagonal", "Equivalent Rect Short Side (Feret)", "Average Horiz. Segment Length", "Average Vert. Segment Length", "Hydraulic Radius", "Waddel Disk Diameter", "-", "Area", "Holes' Area", "Particle & Holes' Area", "Convex Hull Area", "Image Area", "-", "Number of Holes", "Number of Horiz. Segments", "Number of Vert. Segments", "-", "Orientation", "Max Feret Diameter Orientation", "-", "% Area/Image Area", "% Area/(Particle & Holes' Area)", "Ratio of Equivalent Ellipse Axes", "Ratio of Equivalent Rect Sides", "-", "Elongation Factor", "Compactness Factor", "Heywood Circularity Factor", "Type Factor", "-", "Sum X", "Sum Y", "Sum XX", "Sum XY", "Sum YY", "Sum XXX", "Sum XXY", "Sum XYY", "Sum YYY", "-", "Moment of Inertia XX", "Moment of Inertia XY", "Moment of Inertia YY", "Moment of Inertia XXX", "Moment of Inertia XXY", "Moment of Inertia XYY", "Moment of Inertia YYY", "Norm. Moment of Inertia XX", "Norm. Moment of Inertia XY", "Norm. Moment of Inertia YY", "Norm. Moment of Inertia XXX", "Norm. Moment of Inertia XXY", "Norm. Moment of Inertia XYY", "Norm. Moment of Inertia YYY", "Hu Moment 1", "Hu Moment 2", "Hu Moment 3", "Hu Moment 4", "Hu Moment 5", "Hu Moment 6", "Hu Moment 7"] ("Pixel Measurements")
            w526 = 1  # Number of Erosion
            w528 = T10 0 items=["Grayscale (U8)", "Grayscale (I16)", "Grayscale (SGL)", "Complex (CSG)", "RGB (U32)", "HSL (U32)", "RGB (U64)", "Grayscale (U16)"] ("Image Type")
            w537 = T10 1 items=["Grayscale (U8)", "Grayscale (I16)", "Grayscale (SGL)", "Complex (CSG)", "RGB (U32)", "HSL (U32)", "RGB (U64)", "Grayscale (U16)"] ("Image Type")
            # "remove small particles"
            n337 = local write "got copy"(TRUE) -> ()
            n338 = local read "LUT1"() -> (w527:cluster{u16, u16})
            n339 = Unbundle(w527) -> (→"lower":u16, →"upper":u16)
            n340 = call "IMAQ Create"("Image Name"="image copy", "Image Type"=w537) -> ("New Image"=w536:T3)  [unwired: 3 in, 1 out]
            n341 = local read "Image"() -> (w532:T3)
            n342 = call "IMAQ Copy"("Image Dst"=w536, "Image Src"=w532) -> ("Image Dst Out"=w531:T3)  [unwired: 4 in, 1 out]
            "temp copy" <- w531
            n343 = call "IMAQ Threshold"("Range"=w527, "Image Src"=w531) -> ("Image Dst Out"=w530:T3)  [unwired: 4 in, 5 out]
            n344 = call "IMAQ Histograph"("Image"=w531) -> ("Mean Value"=→"Mean Value":sgl, "Histogram Graph"=→"Histogram Graph":T6)  [unwired: 7 in, 2 out]
            n345 = call "IMAQ Cast Image"("Image Type"=w528, "Image Src"=w530) -> ("Image Dst Out"=w529:T3)  [unwired: 8 in, 1 out]
            n346 = call "IMAQ FillHole"("Image Src"=w529) -> ("Image Dst Out"=w515:T3)  [unwired: 3 in, 3 out]
            n347 = disable-structure shown="Disabled" {
              disable-tunnel: w515 -> [w540 _]
              disable-tunnel: [w539 _] -> _
              frame Disabled {
                n348 = call "IMAQ RejectBorder"("Image Src"=w540) -> ("Image Dst Out"=w539:T3)  [unwired: 3 in, 3 out]
              }
              frame Enabled {
              }
            }
            n349 = call "IMAQ RemoveParticle"("Number of Erosion"=w526, "Image Src"=w515) -> ("Image Dst Out"=w522:T3)  [unwired: 5 in, 4 out]
            n350 = call "IMAQ Particle Analysis"("Pixel Measurements"=w525, "Image"=w522) -> ("Particle Measurements (Pixels)"=w517:dbl[][], "Image Out (duplicate)"=w524:T3, "Number of Particles"=→"Number \nof Particles":i32)  [unwired: 4 in, 3 out]
            "Reference Rectangles" <- w517
            n351 = for {
              tunnel: [w541] -> w518
              tunnel: w524 -> [w549]
              tunnel: w517 -> [w547] mode=indexing
              tunnel: T2 {"Left"=0, "Top"=0, "Right"=0, "Bottom"=0} ("Rectangle") -> [w548]
              (unwired) 0.0 ("Rotation")
              n352 = Index Array(array=w547) -> (element #1=w545:dbl, element #2=w544:dbl, element #3=w543:dbl, element #4=w542:dbl)  [unwired: 4 in]
              n353 = Bundle By Name(cluster=w548, "Left"=w545, "Top"=w544, "Right"=w543, "Bottom"=w542) -> (w546:T2)
              n354 = call "IMAQ Overlay Rectangle"("Color"=u32 3407634 ("Text Color (black)"), "Rectangle"=w546, "Image"=w549) -> ("Image Out"=w541:T3)  [unwired: 7 in, 1 out]
            }
            n355 = local write "Reference Screen"(w518) -> ()
            n356 = property on="Reference Screen" class="ImageControl"("Palette Type"=w516) -> ()  [unwired: 2 in, 2 out]
          }
        }
      }
      event "Reference Screen": Mouse Move; "Reference Screen": Mouse Enter; "Reference Screen": Mouse Up; "Reference Screen": Mouse Down {
        n357 = event-data() -> ()  [unwired: 1 in, 3 out]
        n358 = local read "Reference Screen"() -> (w555:T3)
        n359 = invoke on="Reference Screen" class="ImageControl" method="Get Last Event"() -> ("Type"=w553:i32, "Tool"=w552:i32, "Coordinates"=w551:i32[])  [unwired: 8 in, 5 out]
        "Coordinates" <- w551
        n360 = local read "Reference Rectangles"() -> (w554:dbl[][])
        n361 = case shown="1" w553 {
          tunnel: w552 -> [_ w559]
          tunnel: w551 -> [_ w558]
          tunnel: w555 -> [_ w557]
          tunnel: w554 -> [_ w556]
          frame 0, Default {
          }
          frame 1 {
            n362 = case shown="2" w559 {
              tunnel: w558 -> [_ w584]
              tunnel: w557 -> [_ w583]
              tunnel: w556 -> [_ w581]
              frame 0, Default {
              }
              frame 2 {
                w573 = u32 1 items=["Grayscale", "Binary", "Gradient", "Rainbow", "Temperature", "User Defined"] ("Palette:Palette Type")
                n363 = Index Array(array=w584, index #1=0 ("index")) -> (element #1=w580:i32, element #2=w579:i32)  [unwired: 1 in]
                n364 = property on="Reference Screen" class="ImageControl"("Palette Type"=w573) -> ()  [unwired: 2 in, 2 out]
                n365 = Bundle(w580, w579) -> (w582:cluster{i32, i32})  [unwired: 1 in]
                n366 = for {
                  tunnel: w581 -> [w608] mode=indexing
                  tunnel: w580 -> [w607]
                  tunnel: w579 -> [w602]
                  shift-right: [w599] -> w572
                  shift-left: 0.0 -> [w598]
                  shift-right: [w595] -> w564
                  shift-left: 0.0 ("Numeric") -> [w594]
                  shift-right: [w592] -> w567
                  shift-left: 0.0 ("Numeric") -> [w591]
                  shift-right: [w589] -> w560
                  shift-left: 0.0 ("Numeric") -> [w588]
                  n367 = Index Array(array=w608) -> (element #1=w597:dbl, element #2=w596:dbl, element #3=w593:dbl, element #4=w590:dbl)  [unwired: 4 in]
                  n368 = Greater Or Equal?(x=w607, y=w597) -> (x >= y?=w606:bool)
                  n369 = Less Or Equal?(x=w607, y=w593) -> (x <= y?=w605:bool)
                  n370 = Less Or Equal?(x=w602, y=w590) -> (x <= y?=w604:bool)
                  n371 = Greater Or Equal?(x=w602, y=w596) -> (x >= y?=w603:bool)
                  n372 = And(x=w606, y=w605) -> (x .and. y?=w601:bool)
                  n373 = And(x=w604, y=w603) -> (x .and. y?=w600:bool)
                  n374 = And(x=w601, y=w600) -> (x .and. y?=w587:bool)
                  n375 = Select(t=w597, s=w587, f=w598) -> (s? t:f=w599:dbl)
                  n376 = Select(t=w596, s=w587, f=w594) -> (s? t:f=w595:dbl)
                  n377 = Select(t=w593, s=w587, f=w591) -> (s? t:f=w592:dbl)
                  n378 = Select(t=w590, s=w587, f=w588) -> (s? t:f=w589:dbl)
                }
                "Left" <- w572
                "Top" <- w564
                "Right" <- w567
                "Bottom" <- w560
                n379 = call "IMAQ Overlay Points"("Color"=u32 16860 ("Text Color (black)"), "Point"=w582, "Image"=w583) -> ("Image Out"=w574:T3)  [unwired: 7 in, 1 out]
                n380 = local write "Reference Screen"(w574) -> ()
                n381 = To Unsigned Word Integer(number=w567) -> (unsigned 16bit integer=w569:u16)
                n382 = To Unsigned Word Integer(number=w560) -> (unsigned 16bit integer=w563:u16)
                n383 = To Unsigned Word Integer(number=w572) -> (unsigned 16bit integer=w571:u16)
                n384 = To Unsigned Word Integer(number=w564) -> (unsigned 16bit integer=w566:u16)
                n385 = Add(x=w569, y="Boundary") -> (x+y=→"Ref Right":u16)
                n386 = Add(x=w563, y="Boundary") -> (x+y=→"Ref Bottom":u16)
                n387 = Subtract(x=w571, y="Boundary") -> (x-y=→"Ref Left":u16)
                n388 = Subtract(x=w566, y="Boundary") -> (x-y=→"RefTop":u16)
              }
            }
          }
        }
      }
      event "Show Dendrties": Value Change {
        n389 = event-data() -> ()  [unwired: 1 in, 5 out]
        n390 = local read "Show Dendrties"() -> (w609:bool)
        n391 = case shown="True" w609 {
          frame False {
            n392 = local read "Reference Screen"() -> (w611:T3)
            n393 = call "IMAQ Clear Overlay"("Image"=w611) -> ("error out"=w610:errorcluster)  [unwired: 9 in, 1 out]
            n394 = invoke on="Reference Screen" class="ImageControl" method="Clear ROI"(error in=w610) -> ()  [unwired: 2 in, 3 out]
          }
          frame True {
            w627 = 0.0  # max horizontal
            w628 = 0.0  # max vertical
            w644 = T15[] [4, 5, 6, 7] items=["Center of Mass X", "Center of Mass Y", "First Pixel X", "First Pixel Y", "Bounding Rect Left", "Bounding Rect Top", "Bounding Rect Right", "Bounding Rect Bottom", "Max Feret Diameter Start X", "Max Feret Diameter Start Y", "Max Feret Diameter End X", "Max Feret Diameter End Y", "Max Horiz. Segment Length Left", "Max Horiz. Segment Length Right", "Max Horiz. Segment Length Row", "-", "Bounding Rect Width", "Bounding Rect Height", "Bounding Rect Diagonal", "Perimeter", "Convex Hull Perimeter", "Holes' Perimeter", "Max Feret Diameter", "Equivalent Ellipse Major Axis", "Equivalent Ellipse Minor Axis", "Equivalent Ellipse Minor Axis (Feret)", "Equivalent Rect Long Side", "Equivalent Rect Short Side", "Equivalent Rect Diagonal", "Equivalent Rect Short Side (Feret)", "Average Horiz. Segment Length", "Average Vert. Segment Length", "Hydraulic Radius", "Waddel Disk Diameter", "-", "Area", "Holes' Area", "Particle & Holes' Area", "Convex Hull Area", "Image Area", "-", "Number of Holes", "Number of Horiz. Segments", "Number of Vert. Segments", "-", "Orientation", "Max Feret Diameter Orientation", "-", "% Area/Image Area", "% Area/(Particle & Holes' Area)", "Ratio of Equivalent Ellipse Axes", "Ratio of Equivalent Rect Sides", "-", "Elongation Factor", "Compactness Factor", "Heywood Circularity Factor", "Type Factor", "-", "Sum X", "Sum Y", "Sum XX", "Sum XY", "Sum YY", "Sum XXX", "Sum XXY", "Sum XYY", "Sum YYY", "-", "Moment of Inertia XX", "Moment of Inertia XY", "Moment of Inertia YY", "Moment of Inertia XXX", "Moment of Inertia XXY", "Moment of Inertia XYY", "Moment of Inertia YYY", "Norm. Moment of Inertia XX", "Norm. Moment of Inertia XY", "Norm. Moment of Inertia YY", "Norm. Moment of Inertia XXX", "Norm. Moment of Inertia XXY", "Norm. Moment of Inertia XYY", "Norm. Moment of Inertia YYY", "Hu Moment 1", "Hu Moment 2", "Hu Moment 3", "Hu Moment 4", "Hu Moment 5", "Hu Moment 6", "Hu Moment 7"] ("Pixel Measurements")
            w646 = T10 0 items=["Grayscale (U8)", "Grayscale (I16)", "Grayscale (SGL)", "Complex (CSG)", "RGB (U32)", "HSL (U32)", "RGB (U64)", "Grayscale (U16)"] ("Image Type")
            w647 = u32 1 items=["Grayscale", "Binary", "Gradient", "Rainbow", "Temperature", "User Defined"] ("Palette:Palette Type")
            w652 = T10 1 items=["Grayscale (U8)", "Grayscale (I16)", "Grayscale (SGL)", "Complex (CSG)", "RGB (U32)", "HSL (U32)", "RGB (U64)", "Grayscale (U16)"] ("Image Type")
            n395 = call "IMAQ Create"("Image Name"="image copy", "Image Type"=w652) -> ("New Image"=w651:T3)  [unwired: 3 in, 1 out]
            n396 = local read "Image"() -> (w650:T3)
            n397 = local read "LUT1"() -> (w648:cluster{u16, u16})
            n398 = call "IMAQ Copy"("Image Dst"=w651, "Image Src"=w650) -> ("Image Dst Out"=w649:T3)  [unwired: 4 in, 1 out]
            n399 = call "IMAQ Threshold"("Range"=w648, "Image Src"=w649) -> ("Image Dst Out"=w614:T3)  [unwired: 4 in, 5 out]
            n400 = call "IMAQ Cast Image"("Image Type"=w646, "Image Src"=w614) -> ("Image Dst Out"=w613:T3)  [unwired: 8 in, 1 out]
            n401 = call "IMAQ FillHole"("Image Src"=w613) -> ("Image Dst Out"=w612:T3)  [unwired: 5 in, 1 out]
            n402 = call "IMAQ RemoveParticle"("Number of Erosion"=1, "Image Src"=w612) -> ("Image Dst Out"=w641:T3)  [unwired: 5 in, 4 out]
            n403 = call "IMAQ Separation"("Nb of Erosion"=1, "Image Src"=w641) -> ("Image Dst Out"=w638:T3)  [unwired: 8 in, 1 out]
            n404 = call "IMAQ RemoveParticle"("Low Pass/High Pass (Low)"=TRUE, "Number of Erosion"=8, "Image Src"=w638) -> ("Image Dst Out"=w636:T3)  [unwired: 4 in, 4 out]
            n405 = disable-structure shown="Disabled" {
              disable-tunnel: w612 -> [w686 _]
              disable-tunnel: w636 -> [w685 _]
              disable-tunnel: [w684 _] -> _
              frame Disabled {
                w677 = T10 0 items=["Grayscale (U8)", "Grayscale (I16)", "Grayscale (SGL)", "Complex (CSG)", "RGB (U32)", "HSL (U32)", "RGB (U64)", "Grayscale (U16)"] ("Image Type")
                w682 = T10 0 items=["Grayscale (U8)", "Grayscale (I16)", "Grayscale (SGL)", "Complex (CSG)", "RGB (U32)", "HSL (U32)", "RGB (U64)", "Grayscale (U16)"] ("Image Type")
                n406 = call "IMAQ Create"("Image Name"="untitled", "Image Type"=w682) -> ("New Image"=w680:T3)  [unwired: 3 in, 1 out]
                n407 = call "IMAQ Create"("Image Name"="untitled1", "Image Type"=w677) -> ("New Image"=w676:T3)  [unwired: 3 in, 1 out]
                n408 = call "IMAQ Copy"("Image Dst"=w676, "Image Src"=w686) -> ("Image Dst Out"=w675:T3)  [unwired: 4 in, 1 out]
                n409 = call "IMAQ RemoveParticle"("Number of Erosion"=6, "Image Src"=w675) -> ("Image Dst Out"=w679:T3)  [unwired: 5 in, 4 out]
                n410 = call "IMAQ Subtract"("Image Src A"=w685, "Image Dst"=w680, "Image Src B"=w679) -> ("Image Dst Out"=w684:T3)  [unwired: 4 in, 1 out]
              }
              frame Enabled {
              }
            }
            n411 = call "IMAQ RejectBorder"("Image Src"=w636) -> ("Image Dst Out"=w634:T3)  [unwired: 5 in, 1 out]
            n412 = call "IMAQ Morphology"("Structuring Element"=i32[][] [[0, 1, 0], [0, 1, 0], [0, 1, 0]], "Operation"=T14."Dilate", "Image Src"=w634) -> ("Image Dst Out"=w631:T3)  [unwired: 7 in, 1 out]
            n413 = call "IMAQ RemoveParticle"("Number of Erosion"=2, "Image Src"=w631) -> ("Image Dst Out"=w630:T3)  [unwired: 5 in, 4 out]
            n414 = call "IMAQ Particle Analysis"("Pixel Measurements"=w644, "Image"=w630) -> ("Particle Measurements (Pixels)"=w629:dbl[][], "Image Out (duplicate)"=w643:T3)  [unwired: 4 in, 4 out]
            n415 = for {
              tunnel: [w688] -> w623
              tunnel: w643 -> [w696]
              tunnel: w629 -> [w694] mode=indexing
              tunnel: T2 {"Left"=0, "Top"=0, "Right"=0, "Bottom"=0} ("Rectangle") -> [w695]
              tunnel: [w687] -> w616
              (unwired) 0.0 ("Rotation")
              n416 = Index Array(array=w694) -> (element #1=w692:dbl, element #2=w691:dbl, element #3=w690:dbl, element #4=w689:dbl)  [unwired: 4 in]
              n417 = Bundle By Name(cluster=w695, "Left"=w692, "Top"=w691, "Right"=w690, "Bottom"=w689) -> (w693:T2)
              n418 = call "IMAQ Overlay Rectangle"("Color"=u32 3407634 ("Text Color (black)"), "Rectangle"=w693, "Image"=w696) -> ("error out"=w687:errorcluster, "Image Out"=w688:T3)  [unwired: 7 in]
            }
            n419 = for {
              tunnel: w629 -> [w674] mode=indexing
              shift-right: [w669] -> _
              shift-left: w628 -> [w670]
              shift-right: [w658] -> _
              shift-left: w627 -> [w659]
              tunnel: T2 {"Left"=0, "Top"=0, "Right"=0, "Bottom"=0} ("Rectangle") -> [w664]
              shift-right: [w662] -> w622
              shift-left: T2 {"Left"=0, "Top"=0, "Right"=0, "Bottom"=0} ("Rectangle") -> [w661]
              shift-right: [w655] -> w619
              shift-left: T2 {"Left"=0, "Top"=0, "Right"=0, "Bottom"=0} ("Rectangle") -> [w654]
              n420 = Index Array(array=w674) -> (element #1=w668:dbl, element #2=w667:dbl, element #3=w666:dbl, element #4=w665:dbl)  [unwired: 4 in]
              n421 = Subtract(x=w665, y=w667) -> (x-y=w672:dbl)
              "height" <- w672
              n422 = Subtract(x=w666, y=w668) -> (x-y=w673:dbl)
              "width" <- w673
              n423 = Bundle By Name(cluster=w664, "Left"=w668, "Top"=w667, "Right"=w666, "Bottom"=w665) -> (w656:T2)
              n424 = Divide(x=w672, y=w673) -> (x/y=w671:dbl)
              n425 = Divide(x=w673, y=w672) -> (x/y=w660:dbl)
              n426 = Greater?(x=w660, y=w659) -> (0:w657:bool)
              n427 = Greater?(x=w671, y=w670) -> (0:w663:bool)
              n428 = Select(t=w671, s=w663, f=w670) -> (s? t:f=w669:dbl)
              n429 = Select(t=w660, s=w657, f=w659) -> (s? t:f=w658:dbl)
              n430 = Select(t=w656, s=w663, f=w661) -> (s? t:f=w662:T2)
              n431 = Select(t=w656, s=w657, f=w654) -> (s? t:f=w655:T2)
            }
            "most Verital" <- w622
            "most horizontal" <- w619
            n432 = call "IMAQ Overlay Rectangle"("Color"=u32 16711680, "error in (no error)"=w616, "Rectangle"=w622, "Image"=w623) -> ("error out"=w615:errorcluster, "Image Out"=w620:T3)  [unwired: 6 in]
            n433 = property on="Reference Screen" class="ImageControl"("Palette Type"=w647) -> ()  [unwired: 2 in, 2 out]
            n434 = call "IMAQ Overlay Rectangle"("Color"=u32 16711680, "error in (no error)"=w615, "Rectangle"=w619, "Image"=w620) -> ("Image Out"=w617:T3)  [unwired: 6 in, 1 out]
            n435 = local write "Reference Screen"(w617) -> ()
          }
        }
      }
      event "Find Lines": Value Change {
        n436 = event-data() -> ()  [unwired: 1 in, 5 out]
        n437 = local read "Find Lines"() -> (w698:bool)
        n438 = case shown="True" w698 {
          frame False {
          }
          frame True {
            w704 = u32 1 items=["Grayscale", "Binary", "Gradient", "Rainbow", "Temperature", "User Defined"] ("Palette:Palette Type")
            w705 = T10 0 items=["Grayscale (U8)", "Grayscale (I16)", "Grayscale (SGL)", "Complex (CSG)", "RGB (U32)", "HSL (U32)", "RGB (U64)", "Grayscale (U16)"] ("Image Type")
            w711 = T10 1 items=["Grayscale (U8)", "Grayscale (I16)", "Grayscale (SGL)", "Complex (CSG)", "RGB (U32)", "HSL (U32)", "RGB (U64)", "Grayscale (U16)"] ("Image Type")
            n439 = local read "Reference Screen"() -> (w709:T3)
            n440 = call "IMAQ Create"("Image Name"="image copy", "Image Type"=w711) -> ("New Image"=w710:T3)  [unwired: 3 in, 1 out]
            n441 = call "IMAQ Copy"("Image Dst"=w710, "Image Src"=w709) -> ("Image Dst Out"=w707:T3)  [unwired: 4 in, 1 out]
            n442 = local read "LUT1"() -> (w706:cluster{u16, u16})
            n443 = call "IMAQ Threshold"("Range"=w706, "Image Src"=w707) -> ("Image Dst Out"=w708:T3)  [unwired: 4 in, 5 out]
            n444 = call "IMAQ Cast Image"("Image Type"=w705, "Image Src"=w708) -> ("Image Dst Out"=w700:T3)  [unwired: 8 in, 1 out]
            n445 = call-poly "IMAQ Detect Shapes"("Line Descriptor"=cluster{"Min Length":dbl, "Max Length":dbl} {"Min Length"=5.0, "Max Length"=300.0}, "Image"=w700) -> ("Number of Matches Returned"=→"Number of Matches Returned":i32, "Lines"=w701:T1)  [unwired: 7 in, 1 out]
            "Lines" <- w701
            n446 = property on="Reference Screen" class="ImageControl"("Palette Type"=w704) -> ()  [unwired: 2 in, 2 out]
            n447 = for {
              tunnel: w701 -> [w718] mode=indexing
              tunnel: w700 -> [w717]
              tunnel: [w713] -> w699
              n448 = Unbundle By Name(w718) -> ("Start Point"=w716:cluster{"X":sgl, "Y":sgl}, "End Point"=w715:cluster{"X":sgl, "Y":sgl})  [unwired: 3 out]
              n449 = call "IMAQ Overlay Line"("Color"=u32 14876458, "End Point"=w715, "Start Point"=w716, "Image"=w717) -> ("Image Out"=w713:T3)  [unwired: 6 in, 1 out]
            }
            n450 = local write "Reference Screen"(w699) -> ()
          }
        }
      }
    }
    n451 = Multiply(x="DwelTime", y=u32 4) -> (x*y=→"DwelTime2":u32)
    n452 = local read "GridNumberXY"() -> (w101:i8)
    n453 = local read "POISelect Array"() -> (w124:cluster{"System Array":dbl[], "Boolean":bool}[])
    n454 = local read "GridNumberZ"() -> (w102:i8)
    n455 = Array Size(array=w97) -> (size(s)=w99:i32[])
    n456 = Multiply(x=w108, y=4) -> (x*y=w119:u32)
    n457 = Multiply(x="Length(msec)", y=1000.0) -> (x*y=w122:dbl)
    n458 = Index Array(array=w99, index=0) -> (element=w98:i32)
    n459 = Add(x=w119, y=24) -> (x+y=w117:u32)
    n460 = Compound Arithmetic op=MULTIPLY(w101, w102, w101, w98) -> (w103:i32)
    n461 = Multiply(x=w117, y=w103) -> (x*y=w111:u32)
    n462 = Add(x=w111, y=sgl 0.0) -> (x+y=w110:sgl)
    n463 = Divide(x=w122, y=w110) -> (x/y=w114:dbl)
    n464 = Round To Nearest(number=w114) -> (nearest integer value=w115:dbl)
    n465 = Quotient & Remainder(x=w115, y=2.0) -> (x-y*floor(x/y)=w105:dbl)  [unwired: 1 out]
    n466 = Increment(x=w115) -> (x+1=w106:dbl)
    n467 = Not Equal To 0?(x=w105) -> (x != 0?=w104:bool)
    n468 = Select(t=w106, s=w104, f=w115) -> (s? t:f=w113:dbl)
    n469 = To Long Integer(number=w113) -> (32bit integer=→"No. of cycles":i32)
    "TrigDelay(sec) 2" <- "TrigDelay(sec)"
  }
  n470 = Index Array(array=w18, index=0) -> (element=w13:T3)
  n471 = local write "Image"(w13) -> ()
  n472 = disable-structure shown="Disabled" {
    disable-tunnel: w21 -> [w720 _]
    disable-tunnel: w20 -> [w719 _]
    frame Disabled {
      n473 = case shown="True" w719 {
        tunnel: w720 -> [_ w777]
        frame False {
        }
        frame True {
          (unwired) dbl[] [0.0, 0.0] ("f")
          w729 = dbl[] [-2.0, -1.0]  # XYoffset
          w725 = dbl[] [0.0, 0.0]  # XYoffset
          w776 = 270 ("Angle")
          w780 = dbl[] [5.0, 0.0]  # XYoffset
          w726 = dbl[] [-2.0, 0.0]  # XYoffset
          # "POI2NormXYZ V3.vi"
          # "512"
          # "200"
          n474 = local read "Path"() -> (w736:path)
          n475 = local read "No.ofTrials"() -> (w764:dbl)
          n476 = local read "DwelTime"() -> (w763:u32)
          n477 = local read "TrialDelay"() -> (w762:u32)
          n478 = local read "Objective"() -> (w723:u16)
          n479 = local read "Zplanes"() -> (w734:dbl[])
          n480 = call <vilib>:"Recursive File List.vi"("pattern"="points", "Folder Path"=w736) -> ("Number of Files"=w742:i32, "dup Folder Path"=w741:path)  [unwired: 5 in, 3 out]
          n481 = local read "AOD Parameters"() -> (w730:T5)
          n482 = local read "GridNumberXY"() -> (w769:i8)
          n483 = local read "GridNumberZ"() -> (w768:i8)
          n484 = local read "No. of cycles"() -> (w766:i32)
          n485 = local read "Field of View"() -> (w722:u16)
          n486 = call <vilib>:"Recursive File List.vi"("pattern"="norm_points", "Folder Path"=w736) -> ("Number of Files"=w753:i32, "dup Folder Path"=w754:path)  [unwired: 5 in, 3 out]
          n487 = Increment(x=w742) -> (x+1=w743:i32)
          n488 = Build Path(base path=w736, name or relative path="points.dat") -> (appended path=w738:path)
          n489 = Unbundle By Name(w730) -> ("Nvox"=w724:i16, "Zoom"=w731:i8)
          n490 = Select(t=w780, s="ScanMode", f=w725) -> (s? t:f=w779:dbl[])
          n491 = call <vilib>:"Check if File or Folder Exists.vi"("path"=w738) -> ("file or folder exists?"=w739:bool)  [unwired: 8 in, 2 out]
          n492 = Increment(x=w753) -> (x+1=w752:i32)
          n493 = Build Path(base path=w736, name or relative path="norm_points.dat") -> (appended path=w758:path)
          n494 = Number To Decimal String(number=w743) -> (decimal integer string=w745:string)  [unwired: 1 in]
          n495 = call <vilib>:"Check if File or Folder Exists.vi"("path"=w758) -> ("file or folder exists?"=w759:bool)  [unwired: 8 in, 2 out]
          n496 = Number To Decimal String(number=w752) -> (decimal integer string=w750:string)  [unwired: 1 in]
          n497 = Greater Or Equal?(x=w724, y=i16 300) -> (x >= y?=w728:bool)
          n498 = Select(t=w726, s=w728, f=w729) -> ()  [unwired: 1 out]
          n499 = Concatenate Strings("norm_points" ("pattern"), w750, ".dat" ("string")) -> (w748:string)
          n500 = Concatenate Strings("points" ("pattern"), w745, ".dat" ("string")) -> (w747:string)
          n501 = local read "Nvox"() -> (w767:i32)
          n502 = Bundle By Name(cluster=T4 {"xyz coordinates"=[], "Mx offset"=0.0, "My offset"=0.0, "gridnumberXYout"=0, "gridnumberZout"=0, "NvoxOut"=0, "number of cycles out"=0, "AODfill"=0.0, "No. of Trials"=0.0, "Dwell Time"=0, "Trial Delay"=10000} ("Cluster 2"), "xyz coordinates"="NormalizedXYZ", "Mx offset"=0.0, "My offset"=0.0, "gridnumberXYout"=w769, "gridnumberZout"=w768, "NvoxOut"=w767, "number of cycles out"=w766, "AODfill"=1.0, "No. of Trials"=w764, "Dwell Time"=w763, "Trial Delay"=w762) -> (→"output cluster":T4)
          n503 = Build Path(base path=w754, name or relative path=w748) -> (appended path=w755:path)
          n504 = Build Path(base path=w741, name or relative path=w747) -> (appended path=w737:path)
          n505 = Select(t=w755, s=w759, f=w758) -> (s? t:f=w757:path)
          n506 = Select(t=w737, s=w739, f=w738) -> (s? t:f=w735:path)
          n507 = call-poly <userlib>:"Write To Spreadsheet File-Mod.vi"("2D data"="NormalizedXYZ", "file path (dialog if empty)"=w757) -> ()  [unwired: 8 in, 2 out]
          n508 = call-poly <userlib>:"Write To Spreadsheet File-Mod.vi"("file path (dialog if empty)"=w735) -> ("2D data"=w732:dbl[][])  [unwired: 8 in, 2 out]
        }
      }
    }
    frame Enabled {
    }
  }
  "got copy" <- FALSE
